vi "FA ForceAndMoments.vi"() -> ()   [LabVIEW 2016, in "M1M3SupportEUI_Views.lvlib"]
uses:
  M1M3SupportEUI_Views.lvlib
  Model/Model.lvclass
  Typedefs/FA Data And Events.ctl
  SALLV_m1m3/DataTypes/ForceActuatorData.ctl
  SALLV_m1m3/DataTypes/logevent_ForceActuatorForceWarning.ctl
  SALLV_m1m3/DataTypes/logevent_ForceActuatorInfo.ctl
  SALLV_m1m3/DataTypes/logevent_ForceActuatorState.ctl
  SALLV_m1m3/DataTypes/logevent_ForceActuatorWarning.ctl
  SALLV_m1m3/DataTypes/logevent_AppliedAberrationForces.ctl
  SALLV_m1m3/DataTypes/logevent_AppliedAccelerationForces.ctl
  SALLV_m1m3/DataTypes/logevent_AppliedActiveOpticForces.ctl
  SALLV_m1m3/DataTypes/logevent_AppliedAzimuthForces.ctl
  SALLV_m1m3/DataTypes/logevent_AppliedBalanceForces.ctl
  SALLV_m1m3/DataTypes/logevent_AppliedCylinderForces.ctl
  SALLV_m1m3/DataTypes/logevent_AppliedElevationForces.ctl
  SALLV_m1m3/DataTypes/logevent_AppliedForces.ctl
  SALLV_m1m3/DataTypes/logevent_AppliedOffsetForces.ctl
  SALLV_m1m3/DataTypes/logevent_AppliedStaticForces.ctl
  SALLV_m1m3/DataTypes/logevent_AppliedThermalForces.ctl
  SALLV_m1m3/DataTypes/logevent_AppliedVelocityForces.ctl
  SALLV_m1m3/DataTypes/logevent_RejectedAberrationForces.ctl
  SALLV_m1m3/DataTypes/logevent_RejectedAccelerationForces.ctl
  SALLV_m1m3/DataTypes/logevent_RejectedActiveOpticForces.ctl
  SALLV_m1m3/DataTypes/logevent_RejectedAzimuthForces.ctl
  SALLV_m1m3/DataTypes/logevent_RejectedBalanceForces.ctl
  SALLV_m1m3/DataTypes/logevent_RejectedCylinderForces.ctl
  SALLV_m1m3/DataTypes/logevent_RejectedElevationForces.ctl
  SALLV_m1m3/DataTypes/logevent_RejectedForces.ctl
  SALLV_m1m3/DataTypes/logevent_RejectedOffsetForces.ctl
  SALLV_m1m3/DataTypes/logevent_RejectedStaticForces.ctl
  SALLV_m1m3/DataTypes/logevent_RejectedThermalForces.ctl
  SALLV_m1m3/DataTypes/logevent_RejectedVelocityForces.ctl
  M1M3 Support Events/M1M3 Support Events.lvclass/M1M3 Support Events.ctl
  M1M3 Support Events/M1M3 Support Events.lvclass
  <vilib>/Utility/Data Type/NI_Data Type.lvlib
  SALLV_m1m3/SALLV_m1m3.lvlib
  Typedefs/M1M3SupportEUI_TypeDefs.lvlib
panel:
  out "Any Secondary Axis Following Error Warning":bool
  out "Any Primary Axis Following Error Warning":bool
  out "Any Secondary Axis Measured Force Warning":bool
  out "Any Primary Axis Measured Force Warning":bool
  out "Any Force Warning":bool
  out "Support %":sgl format="%_4f"
  out "Balance Forces Applied":bool
  out "Acceleration Forces Applied":bool
  out "Offset Forces Applied":bool
  out "Aberration Forces Applied":bool
  out "Active Optic Forces Applied":bool
  out "Velocity Forces Applied":bool
  out "Thermal Forces Applied":bool
  out "Azimuth Forces Applied":bool
  out "Elevation Forces Applied":bool
  out "Static Forces Applied":bool
  out "Slew Flag":bool
  out "Any Broadcast Counter Warning":bool
  out "Any ILC Fault":bool
  out "Any Mezzanine Application CRC Missing":bool
  out "Any Mezzanine Application Missing":bool
  out "Any Mezzanine Backup Calibration Error":bool
  out "Any Mezzanine Event Trap Reset":bool
  out "Any Mezzanine Main Calibration Error":bool
  out "Any Mezzanine Current Amp 2 Fault":bool
  out "Any Mezzanine Unique Id CRC Error":bool
  out "Any Mezzanine Current Amp 1 Fault":bool
  out "Any Mezzanine Power Fault":bool
  out "Any Aux Power Fault":bool
  out "Any SSR Power Fault":bool
  out "Any Event Trap Reset":bool
  out "Any Brown Out":bool
  out "Any Watchdog Reset":bool
  out "Any One Wire 2 Mismatch":bool
  out "Any One Wire 1 Mismatch":bool
  out "Any One Wire Missing":bool
  out "Any Application CRC Missing":bool
  out "Any Application Missing":bool
  out "Any Application Type Mismatch":bool
  out "Any Unique Id CRC Error":bool
  out "Any Mezzanine Bootloader Active":bool
  out "Any Mezzanine Error":bool
  out "Any Backup Calibration Error":bool
  out "Any Main Calibration Error":bool
  out "Any Fault Override":bool
  out "Any Minor Fault":bool
  out "Any Major Fault":bool
  out "Any Warning":bool
  out "Timestamp":timestamp
  out "Force Magnitude":sgl format="%_8f"
  out "Mx":sgl format="%_8f"
  out "My":sgl format="%_8f"
  out "Mz":sgl format="%_8f"
  out "Fz":sgl format="%_8f"
  out "Fy":sgl format="%_8f"
  out "Fx":sgl format="%_8f"
  in  "FA Data And Events":T1 {"ForceActuatorData"."Timestamp" format="%#_14f"}
  in  "Data Type":string(combo)
  in  "Model in":refnum<class "Model.lvclass">
  # "FA Errors (with Forces and Moments)"
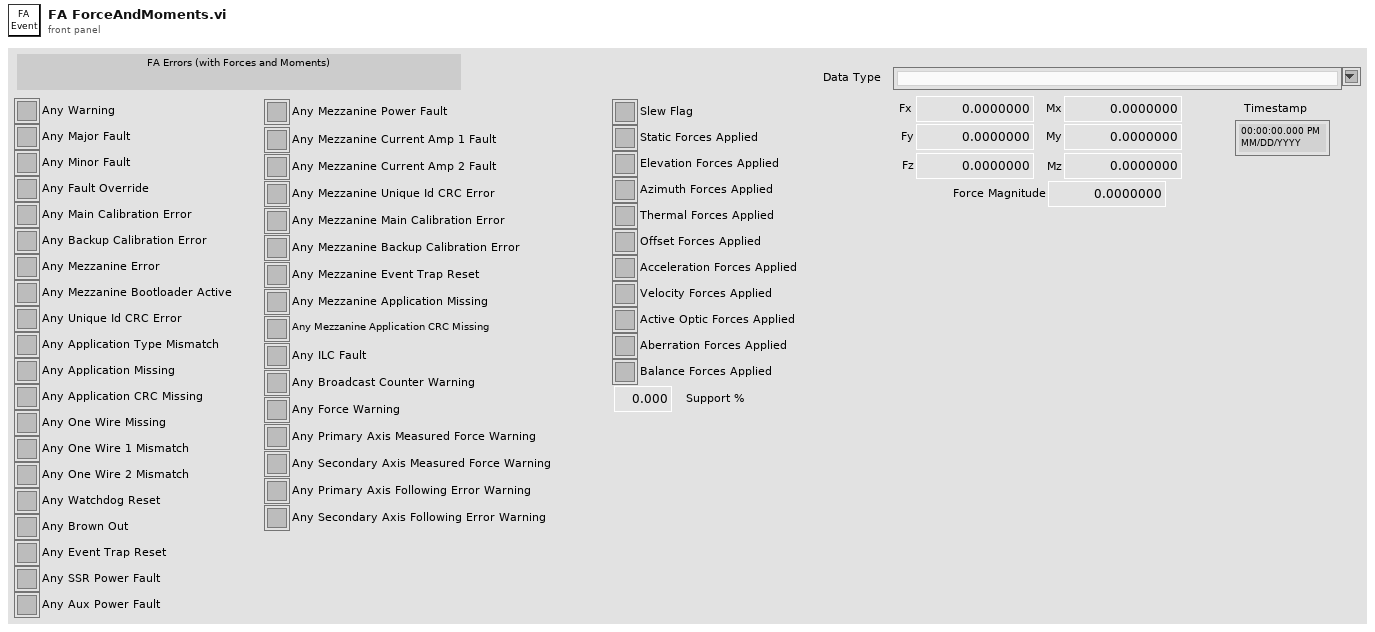
[diagram p1: front panel]
types:
  T1 = typedef "M1M3SupportEUI_TypeDefs.lvlib/FA Data And Events.ctl" = cluster{"ForceActuatorData":T2, "logevent_ForceActuatorForceWarning":T3, "logevent_ForceActuatorInfo":T4, "logevent_ForceActuatorState":T5, "logevent_ForceActuatorWarning":T6, "logevent_AppliedAberrationForces":T7, "logevent_AppliedAccelerationForces":T8, "logevent_AppliedActiveOpticForces":T9, "logevent_AppliedAzimuthForces":T10, "logevent_AppliedBalanceForces":T11, "logevent_AppliedCylinderForces":T12, "logevent_AppliedElevationForces":T13, "logevent_AppliedForces":T14, "logevent_AppliedOffsetForces":T15, "logevent_AppliedStaticForces":T16, "logevent_AppliedThermalForces":T17, "logevent_AppliedVelocityForces":T18, "logevent_RejectedAberrationForces":T19, "logevent_RejectedAccelerationForces":T20, "logevent_RejectedActiveOpticForces":T21, "logevent_RejectedAzimuthForces":T22, "logevent_RejectedBalanceForces":T23, "logevent_RejectedCylinderForces":T24, "logevent_RejectedElevationForces":T25, "logevent_RejectedForces":T26, "logevent_RejectedOffsetForces":T27, "logevent_RejectedStaticForces":T28, "logevent_RejectedThermalForces":T29, "logevent_RejectedVelocityForces":T30}
  T2 = typedef "SALLV_m1m3.lvlib/ForceActuatorData.ctl" = cluster{"Timestamp":dbl, "PrimaryCylinderForce[156]":sgl[], "SecondaryCylinderForce[112]":sgl[], "XForce[12]":sgl[], "YForce[100]":sgl[], "ZForce[156]":sgl[], "Fx":sgl, "Fy":sgl, "Fz":sgl, "Mx":sgl, "My":sgl, "Mz":sgl, "ForceMagnitude":sgl}
  T3 = typedef "SALLV_m1m3.lvlib/logevent_ForceActuatorForceWarning.ctl" = cluster{"Timestamp":dbl, "AnyWarning":bool, "AnyPrimaryAxisMeasuredForceWarning":bool, "PrimaryAxisMeasuredForceWarning[156]":bool[], "AnySecondaryAxisMeasuredForceWarning":bool, "SecondaryAxisMeasuredForceWarning[156]":bool[], "AnyPrimaryAxisFollowingErrorWarning":bool, "PrimaryAxisFollowingErrorWarning[156]":bool[], "AnySecondaryAxisFollowingErrorWarning":bool, "SecondaryAxisFollowingErrorWarning[156]":bool[], "priority":i32}
  T4 = typedef "SALLV_m1m3.lvlib/logevent_ForceActuatorInfo.ctl" = cluster{"Timestamp":dbl, "ReferenceId[156]":i16[], "XDataReferenceId[12]":i16[], "YDataReferenceId[100]":i16[], "ZDataReferenceId[156]":i16[], "ActuatorType[156]":i16[], "ActuatorOrientation[156]":i16[], "ModbusSubnet[156]":i16[], "ModbusAddress[156]":i16[], "XPosition[156]":sgl[], "YPosition[156]":sgl[], "ZPosition[156]":sgl[], "ILCUniqueId[156]":i64[], "ILCApplicationType[156]":i16[], "NetworkNodeType[156]":i16[], "ILCSelectedOptions[156]":i16[], "NetworkNodeOptions[156]":i16[], "MajorRevision[156]":i16[], "MinorRevision[156]":i16[], "ADCScanRate[156]":i16[], "MainPrimaryCylinderCoefficient[156]":sgl[], "MainSecondaryCylinderCoefficient[156]":sgl[], "MainPrimaryCylinderLoadCellOffset[156]":sgl[], "MainSecondaryCylinderLoadCellOffset[156]":sgl[], "MainPrimaryCylinderLoadCellSensitivity[156]":sgl[], "MainSecondaryCylinderLoadCellSensitivity[156]":sgl[], "BackupPrimaryCylinderCoefficient[156]":sgl[], "BackupSecondaryCylinderCoefficient[156]":sgl[], "BackupPrimaryCylinderLoadCellOffset[156]":sgl[], "BackupSecondaryCylinderLoadCellOffset[156]":sgl[], "BackupPrimaryCylinderLoadCellSensitivity[156]":sgl[], "BackupSecondaryCylinderLoadCellSensitivity[156]":sgl[], "MezzaninePrimaryCylinderGain[156]":sgl[], "MezzanineSecondaryCylinderGain[156]":sgl[], "MezzanineUniqueId[156]":i64[], "MezzanineFirmwareType[156]":i16[], "MezzanineMajorRevision[156]":i16[], "MezzanineMinorRevision[156]":i16[], "priority":i32}
  T5 = typedef "SALLV_m1m3.lvlib/logevent_ForceActuatorState.ctl" = cluster{"Timestamp":dbl, "ILCState[156]":i16[], "SlewFlag":bool, "StaticForcesApplied":bool, "ElevationForcesApplied":bool, "AzimuthForcesApplied":bool, "ThermalForcesApplied":bool, "OffsetForcesApplied":bool, "AccelerationForcesApplied":bool, "VelocityForcesApplied":bool, "ActiveOpticForcesApplied":bool, "AberrationForcesApplied":bool, "BalanceForcesApplied":bool, "SupportPercentage":sgl, "priority":i32}
  T6 = typedef "SALLV_m1m3.lvlib/logevent_ForceActuatorWarning.ctl" = cluster{"Timestamp":dbl, "AnyWarning":bool, "AnyMajorFault":bool, "MajorFault[156]":bool[], "AnyMinorFault":bool, "MinorFault[156]":bool[], "AnyFaultOverride":bool, "FaultOverride[156]":bool[], "AnyMainCalibrationError":bool, "MainCalibrationError[156]":bool[], "AnyBackupCalibrationError":bool, "BackupCalibrationError[156]":bool[], "AnyMezzanineError":bool, "MezzanineError[156]":bool[], "AnyMezzanineBootloaderActive":bool, "MezzanineBootloaderActive[156]":bool[], "AnyUniqueIdCRCError":bool, "UniqueIdCRCError[156]":bool[], "AnyApplicationTypeMismatch":bool, "ApplicationTypeMismatch[156]":bool[], "AnyApplicationMissing":bool, "ApplicationMissing[156]":bool[], "AnyApplicationCRCMismatch":bool, "ApplicationCRCMismatch[156]":bool[], "AnyOneWireMissing":bool, "OneWireMissing[156]":bool[], "AnyOneWire1Mismatch":bool, "OneWire1Mismatch[156]":bool[], "AnyOneWire2Mismatch":bool, "OneWire2Mismatch[156]":bool[], "AnyWatchdogReset":bool, "WatchdogReset[156]":bool[], "AnyBrownOut":bool, "BrownOut[156]":bool[], "AnyEventTrapReset":bool, "EventTrapReset[156]":bool[], "AnySSRPowerFault":bool, "SSRPowerFault[156]":bool[], "AnyAuxPowerFault":bool, "AuxPowerFault[156]":bool[], "AnyMezzaninePowerFault":bool, "MezzaninePowerFault[156]":bool[], "AnyMezzanineCurrentAmp1Fault":bool, "MezzanineCurrentAmp1Fault[156]":bool[], "AnyMezzanineCurrentAmp2Fault":bool, "MezzanineCurrentAmp2Fault[156]":bool[], "AnyMezzanineUniqueIdCRCError":bool, "MezzanineUniqueIdCRCError[156]":bool[], "AnyMezzanineMainCalibrationError":bool, "MezzanineMainCalibrationError[156]":bool[], "AnyMezzanineBackupCalibrationError":bool, "MezzanineBackupCalibrationError[156]":bool[], "AnyMezzanineEventTrapReset":bool, "MezzanineEventTrapReset[156]":bool[], "AnyMezzanineApplicationMissing":bool, "MezzanineApplicationMissing[156]":bool[], "AnyMezzanineApplicationCRCMismatch":bool, "MezzanineApplicationCRCMismatch[156]":bool[], "AnyILCFault":bool, "ILCFault[156]":bool[], "AnyBroadcastCounterWarning":bool, "BroadcastCounterWarning[156]":bool[], "priority":i32}
  T7 = typedef "SALLV_m1m3.lvlib/logevent_AppliedAberrationForces.ctl" = cluster{"Timestamp":dbl, "ZForces[156]":sgl[], "Fz":sgl, "Mx":sgl, "My":sgl, "priority":i32}
  T8 = typedef "SALLV_m1m3.lvlib/logevent_AppliedAccelerationForces.ctl" = cluster{"Timestamp":dbl, "XForces[12]":sgl[], "YForces[100]":sgl[], "ZForces[156]":sgl[], "Fx":sgl, "Fy":sgl, "Fz":sgl, "Mx":sgl, "My":sgl, "Mz":sgl, "ForceMagnitude":sgl, "priority":i32}
  T9 = typedef "SALLV_m1m3.lvlib/logevent_AppliedActiveOpticForces.ctl" = cluster{"Timestamp":dbl, "ZForces[156]":sgl[], "Fz":sgl, "Mx":sgl, "My":sgl, "priority":i32}
  T10 = typedef "SALLV_m1m3.lvlib/logevent_AppliedAzimuthForces.ctl" = cluster{"Timestamp":dbl, "XForces[12]":sgl[], "YForces[100]":sgl[], "ZForces[156]":sgl[], "Fx":sgl, "Fy":sgl, "Fz":sgl, "Mx":sgl, "My":sgl, "Mz":sgl, "ForceMagnitude":sgl, "priority":i32}
  T11 = typedef "SALLV_m1m3.lvlib/logevent_AppliedBalanceForces.ctl" = cluster{"Timestamp":dbl, "XForces[12]":sgl[], "YForces[100]":sgl[], "ZForces[156]":sgl[], "Fx":sgl, "Fy":sgl, "Fz":sgl, "Mx":sgl, "My":sgl, "Mz":sgl, "ForceMagnitude":sgl, "priority":i32}
  T12 = typedef "SALLV_m1m3.lvlib/logevent_AppliedCylinderForces.ctl" = cluster{"Timestamp":dbl, "SecondaryCylinderForces[112]":i32[], "PrimaryCylinderForces[156]":i32[], "priority":i32}
  T13 = typedef "SALLV_m1m3.lvlib/logevent_AppliedElevationForces.ctl" = cluster{"Timestamp":dbl, "XForces[12]":sgl[], "YForces[100]":sgl[], "ZForces[156]":sgl[], "Fx":sgl, "Fy":sgl, "Fz":sgl, "Mx":sgl, "My":sgl, "Mz":sgl, "ForceMagnitude":sgl, "priority":i32}
  T14 = typedef "SALLV_m1m3.lvlib/logevent_AppliedForces.ctl" = cluster{"Timestamp":dbl, "XForces[12]":sgl[], "YForces[100]":sgl[], "ZForces[156]":sgl[], "Fx":sgl, "Fy":sgl, "Fz":sgl, "Mx":sgl, "My":sgl, "Mz":sgl, "ForceMagnitude":sgl, "priority":i32}
  T15 = typedef "SALLV_m1m3.lvlib/logevent_AppliedOffsetForces.ctl" = cluster{"Timestamp":dbl, "XForces[12]":sgl[], "YForces[100]":sgl[], "ZForces[156]":sgl[], "Fx":sgl, "Fy":sgl, "Fz":sgl, "Mx":sgl, "My":sgl, "Mz":sgl, "ForceMagnitude":sgl, "priority":i32}
  T16 = typedef "SALLV_m1m3.lvlib/logevent_AppliedStaticForces.ctl" = cluster{"Timestamp":dbl, "XForces[12]":sgl[], "YForces[100]":sgl[], "ZForces[156]":sgl[], "Fx":sgl, "Fy":sgl, "Fz":sgl, "Mx":sgl, "My":sgl, "Mz":sgl, "ForceMagnitude":sgl, "priority":i32}
  T17 = typedef "SALLV_m1m3.lvlib/logevent_AppliedThermalForces.ctl" = cluster{"Timestamp":dbl, "XForces[12]":sgl[], "YForces[100]":sgl[], "ZForces[156]":sgl[], "Fx":sgl, "Fy":sgl, "Fz":sgl, "Mx":sgl, "My":sgl, "Mz":sgl, "ForceMagnitude":sgl, "priority":i32}
  T18 = typedef "SALLV_m1m3.lvlib/logevent_AppliedVelocityForces.ctl" = cluster{"Timestamp":dbl, "XForces[12]":sgl[], "YForces[100]":sgl[], "ZForces[156]":sgl[], "Fx":sgl, "Fy":sgl, "Fz":sgl, "Mx":sgl, "My":sgl, "Mz":sgl, "ForceMagnitude":sgl, "priority":i32}
  T19 = typedef "SALLV_m1m3.lvlib/logevent_RejectedAberrationForces.ctl" = cluster{"Timestamp":dbl, "ZForces[156]":sgl[], "Fz":sgl, "Mx":sgl, "My":sgl, "priority":i32}
  T20 = typedef "SALLV_m1m3.lvlib/logevent_RejectedAccelerationForces.ctl" = cluster{"Timestamp":dbl, "XForces[12]":sgl[], "YForces[100]":sgl[], "ZForces[156]":sgl[], "Fx":sgl, "Fy":sgl, "Fz":sgl, "Mx":sgl, "My":sgl, "Mz":sgl, "ForceMagnitude":sgl, "priority":i32}
  T21 = typedef "SALLV_m1m3.lvlib/logevent_RejectedActiveOpticForces.ctl" = cluster{"Timestamp":dbl, "ZForces[156]":sgl[], "Fz":sgl, "Mx":sgl, "My":sgl, "priority":i32}
  T22 = typedef "SALLV_m1m3.lvlib/logevent_RejectedAzimuthForces.ctl" = cluster{"Timestamp":dbl, "XForces[12]":sgl[], "YForces[100]":sgl[], "ZForces[156]":sgl[], "Fx":sgl, "Fy":sgl, "Fz":sgl, "Mx":sgl, "My":sgl, "Mz":sgl, "ForceMagnitude":sgl, "priority":i32}
  T23 = typedef "SALLV_m1m3.lvlib/logevent_RejectedBalanceForces.ctl" = cluster{"Timestamp":dbl, "XForces[12]":sgl[], "YForces[100]":sgl[], "ZForces[156]":sgl[], "Fx":sgl, "Fy":sgl, "Fz":sgl, "Mx":sgl, "My":sgl, "Mz":sgl, "ForceMagnitude":sgl, "priority":i32}
  T24 = typedef "SALLV_m1m3.lvlib/logevent_RejectedCylinderForces.ctl" = cluster{"Timestamp":dbl, "SecondaryCylinderForces[112]":i32[], "PrimaryCylinderForces[156]":i32[], "priority":i32}
  T25 = typedef "SALLV_m1m3.lvlib/logevent_RejectedElevationForces.ctl" = cluster{"Timestamp":dbl, "XForces[12]":sgl[], "YForces[100]":sgl[], "ZForces[156]":sgl[], "Fx":sgl, "Fy":sgl, "Fz":sgl, "Mx":sgl, "My":sgl, "Mz":sgl, "ForceMagnitude":sgl, "priority":i32}
  T26 = typedef "SALLV_m1m3.lvlib/logevent_RejectedForces.ctl" = cluster{"Timestamp":dbl, "XForces[12]":sgl[], "YForces[100]":sgl[], "ZForces[156]":sgl[], "Fx":sgl, "Fy":sgl, "Fz":sgl, "Mx":sgl, "My":sgl, "Mz":sgl, "ForceMagnitude":sgl, "priority":i32}
  T27 = typedef "SALLV_m1m3.lvlib/logevent_RejectedOffsetForces.ctl" = cluster{"Timestamp":dbl, "XForces[12]":sgl[], "YForces[100]":sgl[], "ZForces[156]":sgl[], "Fx":sgl, "Fy":sgl, "Fz":sgl, "Mx":sgl, "My":sgl, "Mz":sgl, "ForceMagnitude":sgl, "priority":i32}
  T28 = typedef "SALLV_m1m3.lvlib/logevent_RejectedStaticForces.ctl" = cluster{"Timestamp":dbl, "XForces[12]":sgl[], "YForces[100]":sgl[], "ZForces[156]":sgl[], "Fx":sgl, "Fy":sgl, "Fz":sgl, "Mx":sgl, "My":sgl, "Mz":sgl, "ForceMagnitude":sgl, "priority":i32}
  T29 = typedef "SALLV_m1m3.lvlib/logevent_RejectedThermalForces.ctl" = cluster{"Timestamp":dbl, "XForces[12]":sgl[], "YForces[100]":sgl[], "ZForces[156]":sgl[], "Fx":sgl, "Fy":sgl, "Fz":sgl, "Mx":sgl, "My":sgl, "Mz":sgl, "ForceMagnitude":sgl, "priority":i32}
  T30 = typedef "SALLV_m1m3.lvlib/logevent_RejectedVelocityForces.ctl" = cluster{"Timestamp":dbl, "XForces[12]":sgl[], "YForces[100]":sgl[], "ZForces[156]":sgl[], "Fx":sgl, "Fy":sgl, "Fz":sgl, "Mx":sgl, "My":sgl, "Mz":sgl, "ForceMagnitude":sgl, "priority":i32}
  T31 = typedef "M1M3SupportEUI_TypeDefs.lvlib/M1M3 Support Events.ctl" = cluster{"Inclinometer  Data":refnum<user-event>, "IMS Data":refnum<user-event>, "SAL Connected":refnum<user-event>, "Accelerometer Data":refnum<user-event>, "OuterLoop Data":refnum<user-event>, "ErrorCode Event":refnum<user-event>, "InterlockStatus Event":refnum<user-event>, "InterlockWarning Event":refnum<user-event>, "Gyro Data":refnum<user-event>, "HP Actuator Info Event":refnum<user-event>, " FA Info Event":refnum<user-event>, "HP Monitor Info Event":refnum<user-event>, "FA Data":refnum<user-event>, "HP Actuator data":refnum<user-event>, "HP Monitor data":refnum<user-event>, "Air Supply Status Event":refnum<user-event>, "Air Supply Warning Event":refnum<user-event>, "Power Data":refnum<user-event>, "PID Data":refnum<user-event>, "PID Info Event":refnum<user-event>, "Power Status Event":refnum<user-event>, "Power Supply Status Event":refnum<user-event>, "Power Warning Event":refnum<user-event>, "Summary State Event":refnum<user-event>, "Detailed State Event":refnum<user-event>, "FA Force Warning Event":refnum<user-event>, "FA Warning Event":refnum<user-event>, "FA State Event":refnum<user-event>, "Applied AberrationForces Event":refnum<user-event>, "Applied Acceleration Forcces Event":refnum<user-event>, "Applied Azimuth Forces Event":refnum<user-event>, "Applied Active Optic Forces Event":refnum<user-event>, "Applied Balance Forces Event":refnum<user-event>, "Applied Cylinder Forces Event":refnum<user-event>, "Applied Elevation Forces Event":refnum<user-event>, "Applied Forces Event":refnum<user-event>, "Applied Offset Forces Event":refnum<user-event>, "Applied Static Forces Event":refnum<user-event>, "Applied Thermal Forces Event":refnum<user-event>, "Applied Velocity Forces Event":refnum<user-event>, "Rejected Aberration Force Event":refnum<user-event>, "Rejected Acceleration Forces Event":refnum<user-event>, "Rejected Active Optic Forces Event":refnum<user-event>, "Rejected Azimuth Forces Event":refnum<user-event>, "Rejected Balance Forces Event":refnum<user-event>, "Rejected Cylinder Forces Event":refnum<user-event>, "Rejected Elevation Forces Event":refnum<user-event>, "Rejected Forces Event":refnum<user-event>, "Rejected Offset Forces Event":refnum<user-event>, "Rejected Static Forces Event":refnum<user-event>, "Rejected Thermal Forces Event":refnum<user-event>, "Rejected Velocity Forces Event":refnum<user-event>, "Command Rejection Event":refnum<user-event>, "Setting Verions Event":refnum<user-event>, "Settings Applied Event":refnum<user-event>}
  T32 = typedef "NI_Data Type.lvlib/Data Type.ctl" = enum8{"Invalid Type", "Void", "I8", "I16", "I32", "I64", "U8", "U16", "U32", "U64", "Single Float", "Double Float", "Extended Float", "Single Complex", "Double Complex", "Extended Complex", "Enum U8", "Enum U16", "Enum U32", "Enum U64", "Single Float With Unit", "Double Float With Unit", "Extended Float With Unit", "Single Complex with Unit", "Double Complex with Unit", "Extended Complex with Unit", "Boolean", "String", "Path", "Picture", "Tag", "Array", "Cluster", "Variant", "LV Variant", "Waveform", "Timestamp", "Digital Waveform", "Digital Data", "ExpressData", "Refnum", "External Data", "VI", "Poly VI", "LabVIEW Class Instance", "Fixed Point"}
  T33 = enum16{"", "DetailedState_DetailedStates_DisabledState", "DetailedState_DetailedStates_EnabledState", "DetailedState_DetailedStates_FaultState", "DetailedState_DetailedStates_OfflineState", "DetailedState_DetailedStates_StandbyState", "DetailedState_DetailedStates_ParkedState", "DetailedState_DetailedStates_RaisingState", "DetailedState_DetailedStates_ActiveState", "DetailedState_DetailedStates_LoweringState", "DetailedState_DetailedStates_EngineeringState", "DetailedState_DetailedStates_ParkedEngineeringState", "DetailedState_DetailedStates_RaisingEngineeringState", "DetailedState_DetailedStates_ActiveEngineeringState", "DetailedState_DetailedStates_LoweringEngineeringState", "DetailedState_DetailedStates_LoweringFaultState", "DetailedState_DetailedStates_ProfileHardpointCorrectionState"}
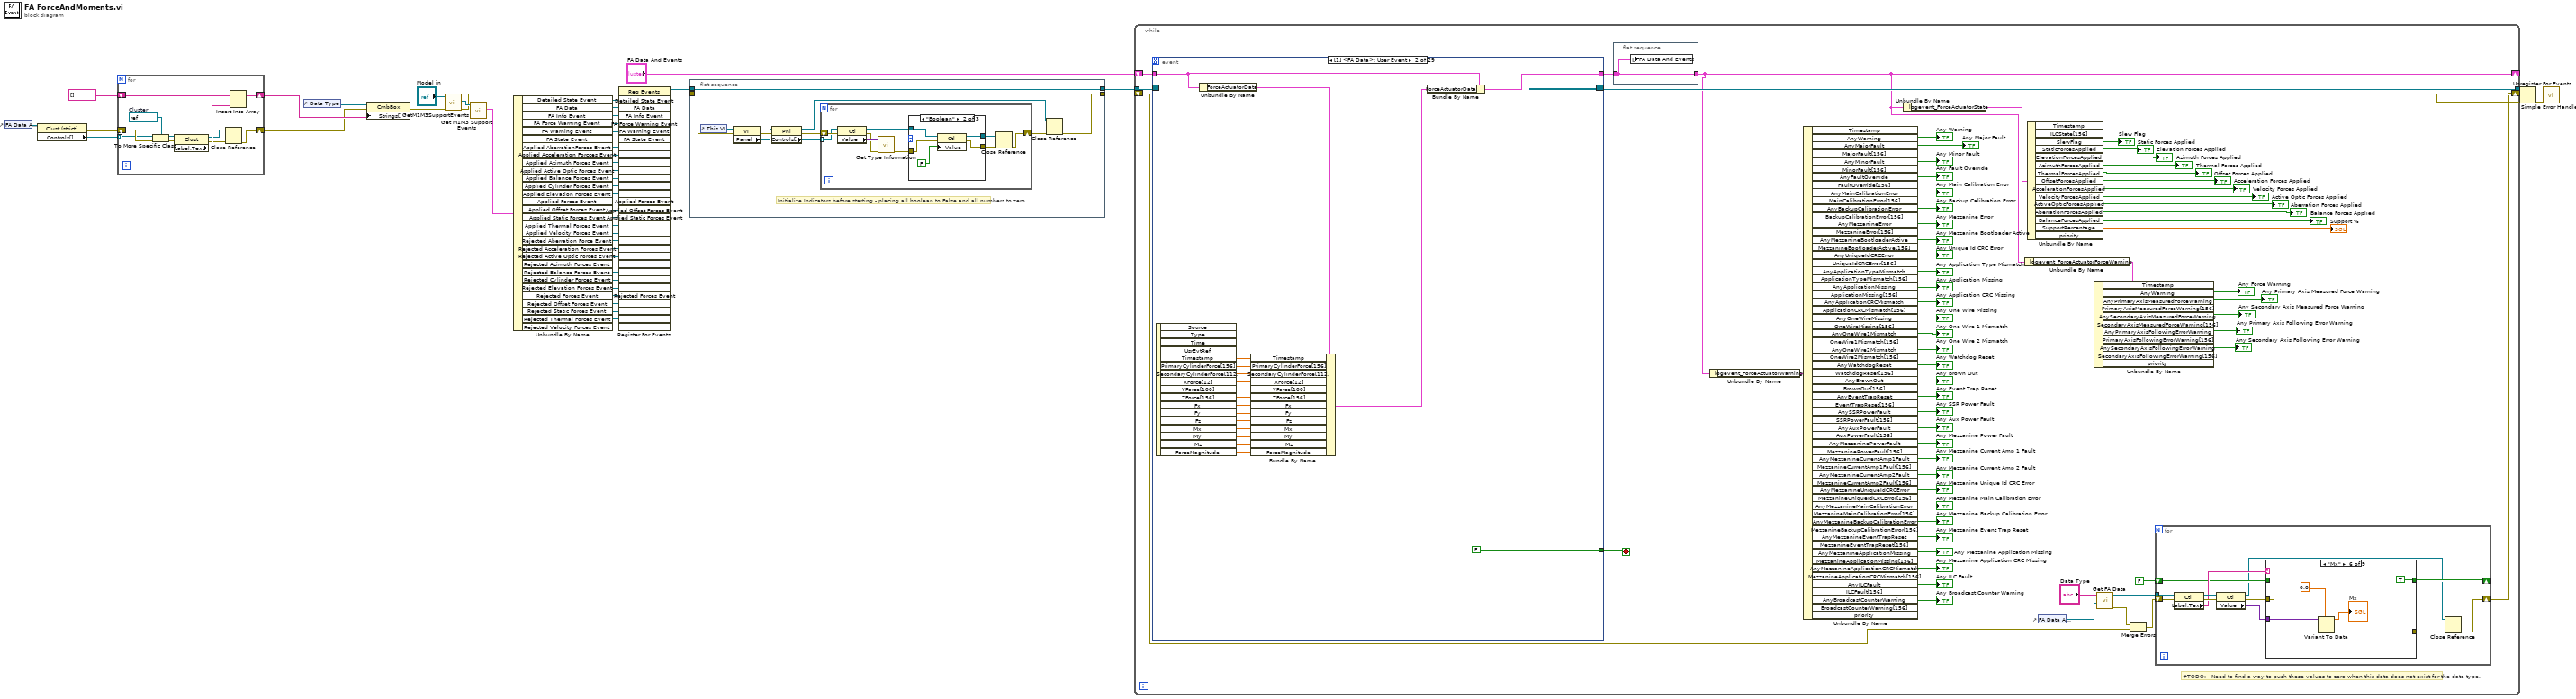
[diagram p0: block diagram]
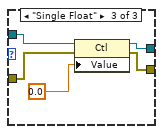
[diagram p3: hidden frame]
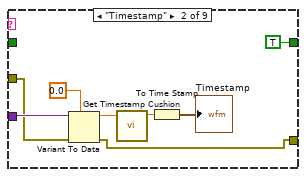
[diagram p5: hidden frame]
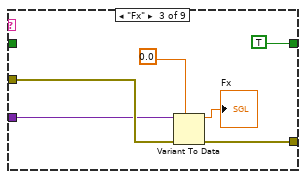
[diagram p6: hidden frame]
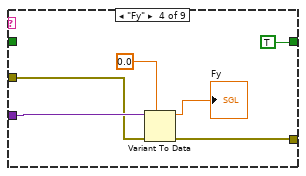
[diagram p7: hidden frame]
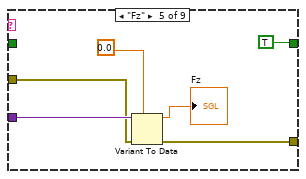
[diagram p8: hidden frame]
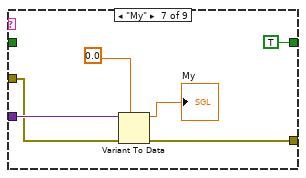
[diagram p9: hidden frame]
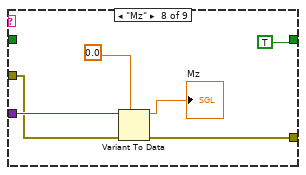
[diagram p10: hidden frame]
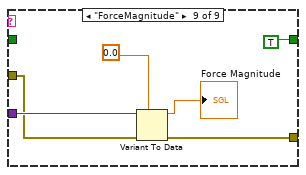
[diagram p11: hidden frame]
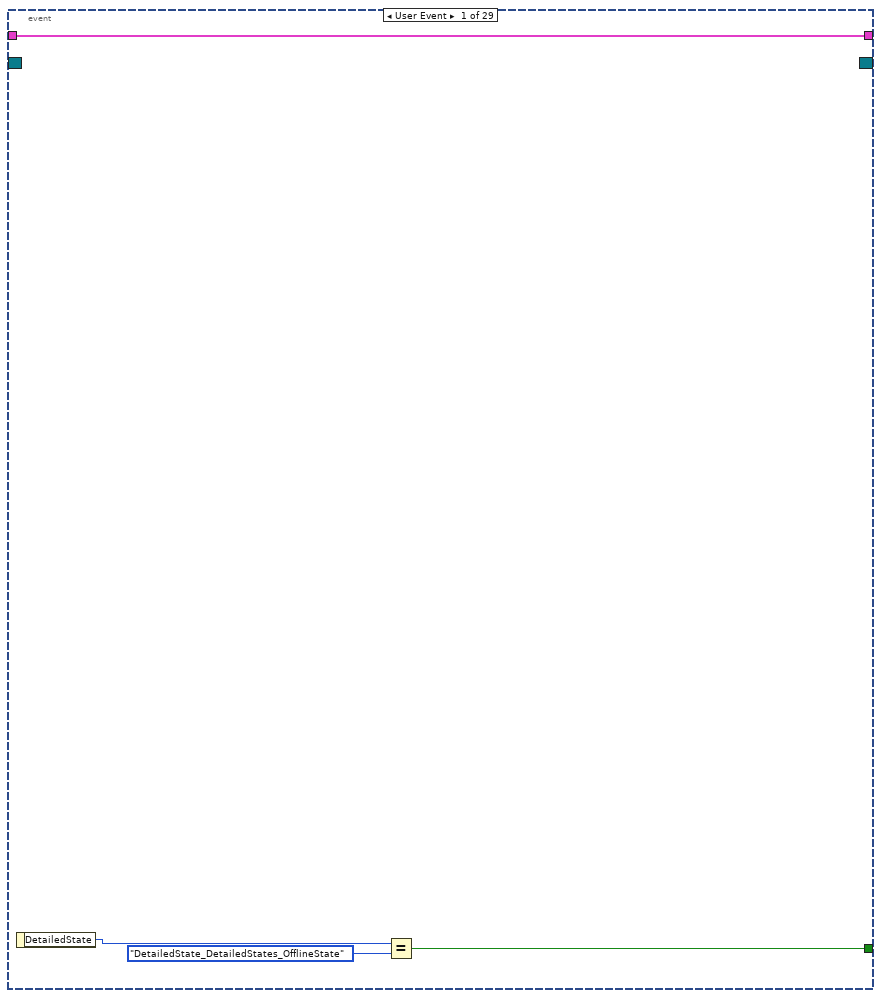
[diagram p12: hidden frame]
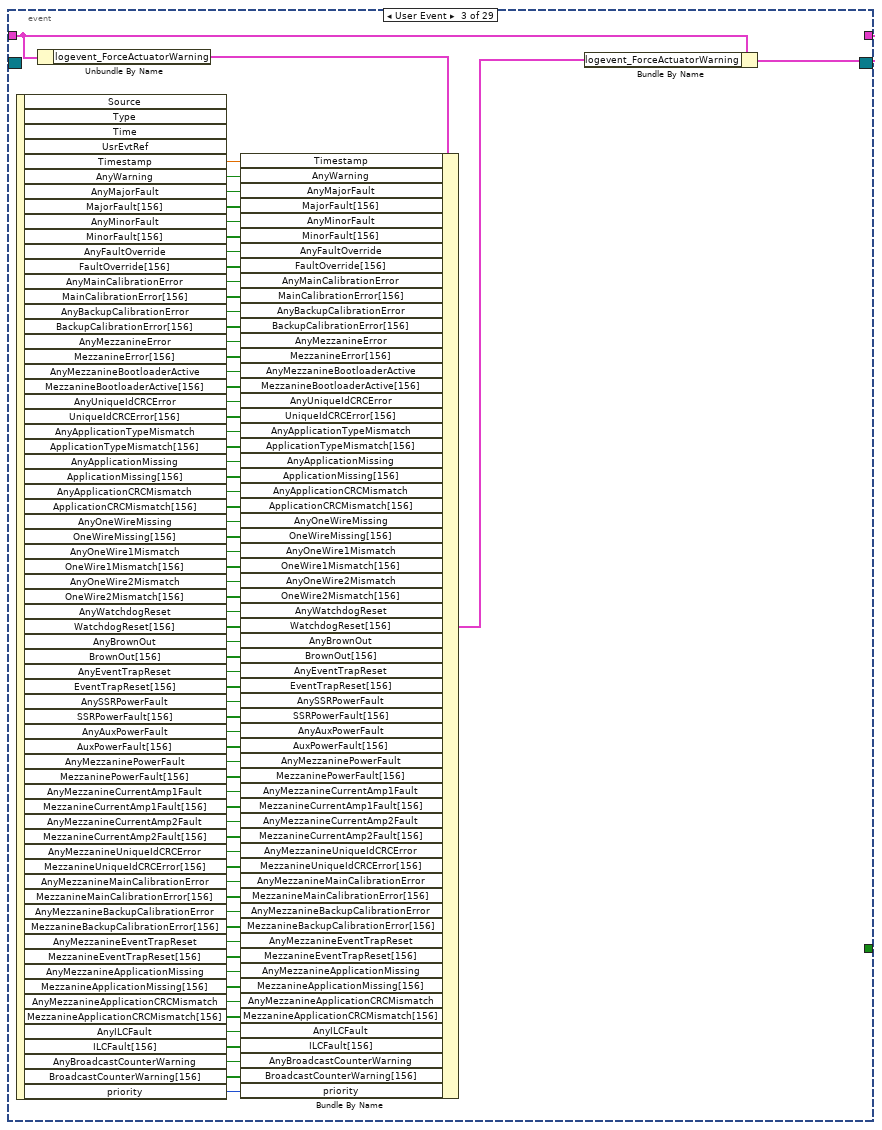
[diagram p13: hidden frame]
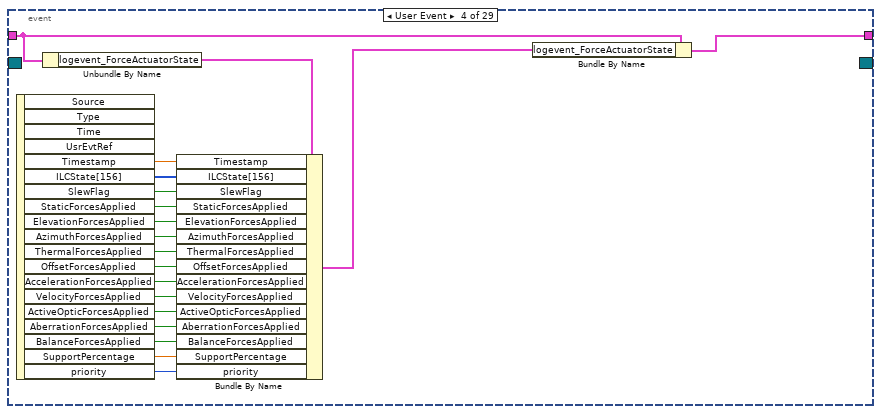
[diagram p14: hidden frame]
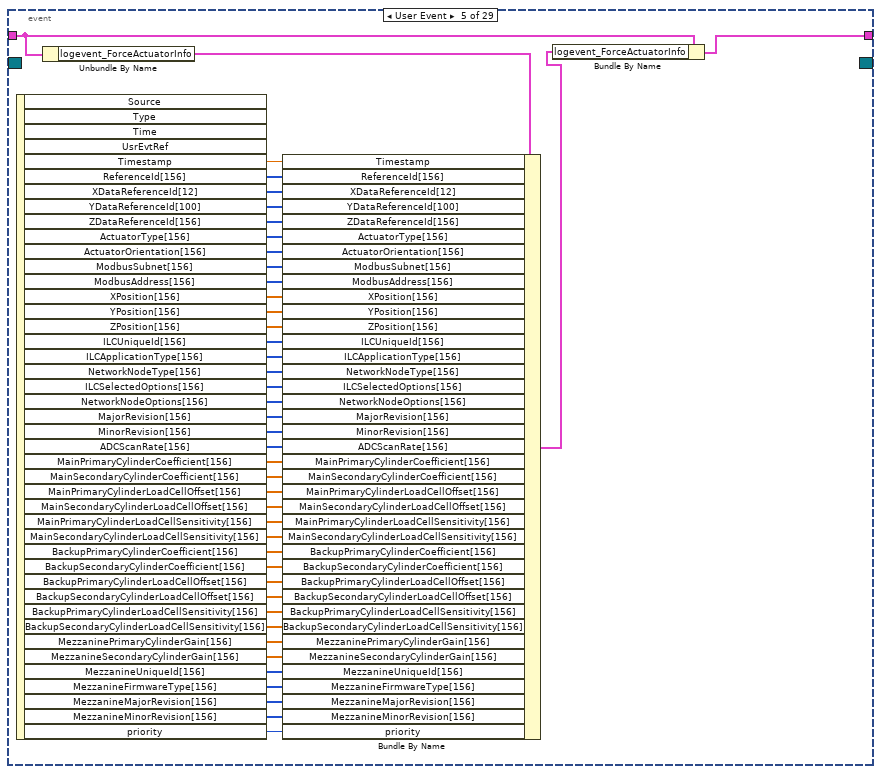
[diagram p15: hidden frame]
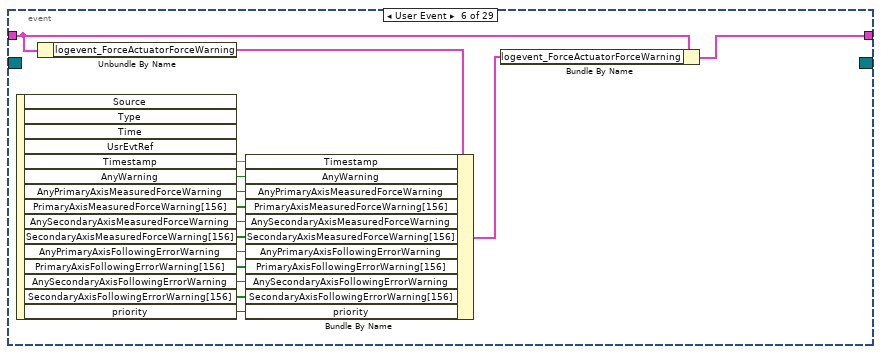
[diagram p16: hidden frame]
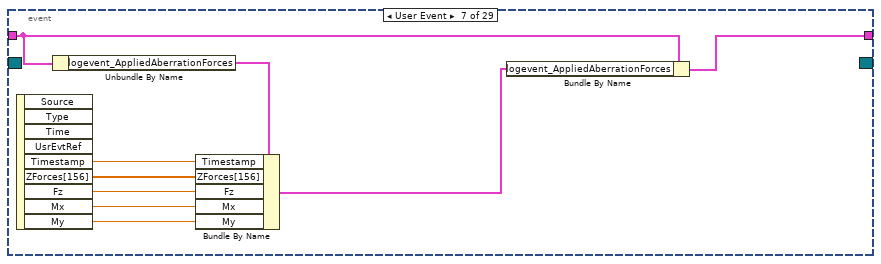
[diagram p17: hidden frame]
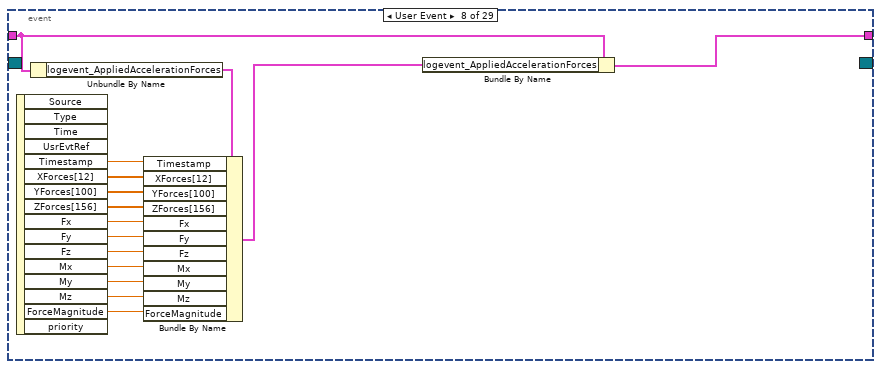
[diagram p18: hidden frame]
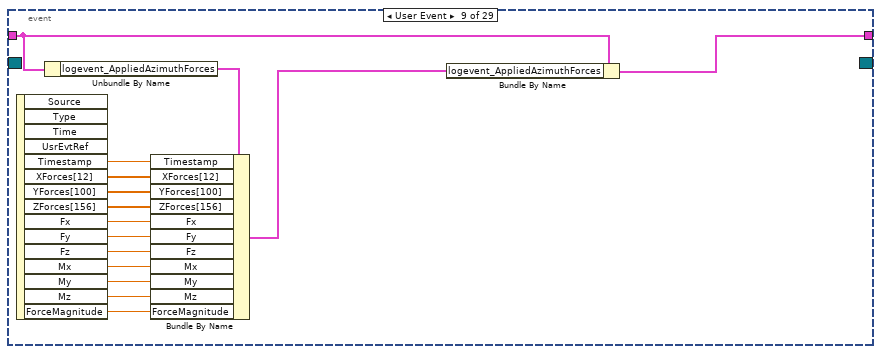
[diagram p19: hidden frame]
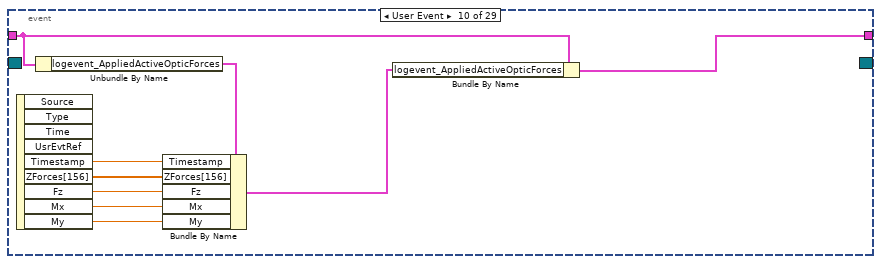
[diagram p20: hidden frame]
diagram:
  n1 = control-ref of="FA Data And Events"() -> (w7:refnum<vi>)
  n2 = property class="Clust (strict)"(reference=w7) -> (error out=w9:errorcluster, "Controls[]"=w10:refnum<vi>[])  [unwired: 1 in, 1 out]
  n3 = for {
    shift-right: [w52] -> w1
    shift-left: w9 -> [w58]
    tunnel: w10 -> [w57] mode=indexing
    shift-right: [w56] -> w8
    shift-left: string[] [] -> [w55]
    w61 = refnum<vi> refnum  # Cluster
    n4 = To More Specific Class(target class=w61, reference=w57, error in=w58) -> (specific class reference=w60:refnum<vi>, error out=w59:errorcluster)
    n5 = property class="Clust"(reference=w60, error in=w59) -> (reference out=w51:refnum<vi>, error out=w53:errorcluster, "Label.Text"=w54:string)
    n6 = Close Reference(reference=w51, error in (no error)=w53) -> (error out=w52:errorcluster)
    n7 = Insert Into Array(array=w55, new element=w54) -> (w56:string[])  [unwired: 1 in]
  }
  n8 = control-ref of="Data Type"() -> (w50:refnum<vi>)
  n9 = property class="CmbBox"(reference=w50, error in=w1, "Strings[]"=w8) -> (error out=w2:errorcluster)  [unwired: 1 out]
  n10 = call "GetM1M3SupportEvents.vi"("error in (no error)"=w2, "Model in"="Model in") -> ("error out"=w17:errorcluster, "M1M3 Support Events out"=w49:refnum<class "M1M3 Support Events.lvclass">)  [unwired: 7 in, 1 out]
  n11 = call "Get M1M3 Support Events.vi"("M1M3 Support Events in"=w49) -> ("M1M3 Support Events"=w16:T31)  [unwired: 9 in, 1 out]
  n12 = Unbundle By Name(w16) -> ("Detailed State Event"=w18:refnum<user-event>, "FA Data"=w19:refnum<user-event>, "FA Info Event"=w20:refnum<user-event>, "FA Force Warning Event"=w21:refnum<user-event>, "FA Warning Event"=w23:refnum<user-event>, "FA State Event"=w22:refnum<user-event>, "Applied AberrationForces Event"=w24:refnum<user-event>, "Applied Acceleration Forcces Event"=w25:refnum<user-event>, "Applied Azimuth Forces Event"=w26:refnum<user-event>, "Applied Active Optic Forces Event"=w27:refnum<user-event>, "Applied Balance Forces Event"=w28:refnum<user-event>, "Applied Cylinder Forces Event"=w29:refnum<user-event>, "Applied Elevation Forces Event"=w30:refnum<user-event>, "Applied Forces Event"=w31:refnum<user-event>, "Applied Offset Forces Event"=w32:refnum<user-event>, "Applied Static Forces Event"=w33:refnum<user-event>, "Applied Thermal Forces Event"=w34:refnum<user-event>, "Applied Velocity Forces Event"=w35:refnum<user-event>, "Rejected Aberration Force Event"=w36:refnum<user-event>, "Rejected Acceleration Forces Event"=w37:refnum<user-event>, "Rejected Active Optic Forces Event"=w38:refnum<user-event>, "Rejected Azimuth Forces Event"=w39:refnum<user-event>, "Rejected Balance Forces Event"=w40:refnum<user-event>, "Rejected Cylinder Forces Event"=w41:refnum<user-event>, "Rejected Elevation Forces Event"=w42:refnum<user-event>, "Rejected Forces Event"=w43:refnum<user-event>, "Rejected Offset Forces Event"=w44:refnum<user-event>, "Rejected Static Forces Event"=w45:refnum<user-event>, "Rejected Thermal Forces Event"=w46:refnum<user-event>, "Rejected Velocity Forces Event"=w47:refnum<user-event>)
  n13 = register-events(error in=w17, w18, w19, w20, w21, w23, w22, w24, w25, w26, w27, w28, w29, w30, w31, w32, w33, w34, w35, w36, w37, w38, w39, w40, w41, w42, w43, w44, w45, w46, w47) -> (reference out=w5:refnum<event-registration>, error out=w4:errorcluster)  [unwired: 1 in]
  n14 = flat-sequence {
    tunnel: [w71] -> w6
    tunnel: w5 -> [w71]
    tunnel: w4 -> [w67]
    tunnel: [w62] -> w3
    frame #0 {
      # "Initialize Indicators before starting - placing all boolean to False and all numbers to zero."
      n15 = control-ref of="This VI"() -> (w70:refnum<vi>)
      n16 = property class="VI"(reference=w70, error in=w67) -> (error out=w69:errorcluster, "Panel"=w68:refnum<vi>)  [unwired: 1 out]
      n17 = property class="Pnl"(reference=w68, error in=w69) -> (reference out=w64:refnum<vi>, error out=w65:errorcluster, "Controls[]"=w66:refnum<vi>[])
      n18 = for {
        tunnel: w66 -> [w80] mode=indexing
        shift-right: [w73] -> w63
        shift-left: w65 -> [w81]
        n19 = property class="Ctl"(reference=w80, error in=w81) -> (reference out=w76:refnum<vi>, error out=w78:errorcluster, "Value"=w79:variant)
        n20 = call <vilib>:"Get Type Information.vi"("error in (no error)"=w78, "Variant"=w79) -> ("error out"=w77:errorcluster, "Type"=w72:T32)  [unwired: 5 in, 3 out]
        n21 = case shown="\"Boolean\"" w72 {
          tunnel: w77 -> [w82 w86 w92]
          tunnel: w76 -> [w83 w88 w93]
          tunnel: [w83 w85 w91] -> w75
          tunnel: [w82 w84 w90] -> w74
          frame "Invalid Type", Default {
          }
          frame "Boolean" {
            n22 = property class="Ctl"(reference=w88, error in=w86, "Value"=FALSE) -> (reference out=w85:refnum<vi>, error out=w84:errorcluster)
          }
          frame "Single Float" {
            n23 = property class="Ctl"(reference=w93, error in=w92, "Value"=sgl 0.0) -> (reference out=w91:refnum<vi>, error out=w90:errorcluster)
          }
        }
        n24 = Close Reference(reference=w75, error in (no error)=w74) -> (error out=w73:errorcluster)
      }
      n25 = Close Reference(reference=w64, error in (no error)=w63) -> (error out=w62:errorcluster)
    }
  }
  n26 = while {
    tunnel: w6 -> [w157]
    tunnel: [w156] -> w15
    shift-right: [w95] -> w14
    shift-left: w3 -> [w96]
    shift-right: [w97] -> _
    shift-left: "FA Data And Events" -> [w158]
    stop <- w155 stop-if-true
    # "#TODO:   Need to find a way to push these values to zero when this data does not exist for the data type."
    n27 = event shown="[1] <FA Data>: User Event" {
      selector: w157 -> [_ _ _ _ _ _ _ _ _ _ _ _ _ _ _ _ _ _ _ _ _ _ _ _ _ _ _ _ _]
      dyn-events: [_ _ _ _ _ _ _ _ _ _ _ _ _ _ _ _ _ _ _ _ _ _ _ _ _ _ _ _ _] -> w156
      timeout: _ -> [_ _ _ _ _ _ _ _ _ _ _ _ _ _ _ _ _ _ _ _ _ _ _ _ _ _ _ _ _]
      tunnel: [w227 FALSE _ _ _ _ _ _ _ _ _ _ _ _ _ _ _ _ _ _ _ _ _ _ _ _ _ _ _] -> w155
      tunnel: w158 -> [w226 w237 w279 w327 w334 w382 w392 w401 w416 w431 w440 w455 w462 w477 w492 w507 w521 w537 w552 w561 w576 w585 w600 w615 w622 w637 w652 w667 w682]
      tunnel: [w226 w235 w278 w325 w333 w381 w390 w399 w414 w429 w438 w453 w460 w475 w490 w505 w520 w535 w550 w559 w574 w583 w598 w613 w620 w635 w650 w665 w680] -> w154
      event User Event {
        n28 = event-data() -> ("DetailedState"=w225:T33)  [unwired: 1 in]
        n29 = Equal?(x=w225, y=T33."DetailedState_DetailedStates_OfflineState") -> (x = y?=w227:bool)
      }
      event User Event {
        n30 = event-data() -> ("Timestamp"=w239:dbl, "PrimaryCylinderForce[156]"=w244:sgl[], "SecondaryCylinderForce[112]"=w243:sgl[], "XForce[12]"=w242:sgl[], "YForce[100]"=w241:sgl[], "ZForce[156]"=w240:sgl[], "Fx"=w234:sgl, "Fy"=w233:sgl, "Fz"=w232:sgl, "Mx"=w231:sgl, "My"=w230:sgl, "Mz"=w229:sgl, "ForceMagnitude"=w228:sgl)  [unwired: 1 in, 4 out]
        n31 = Unbundle By Name(w237) -> ("ForceActuatorData"=w238:T2)
        n32 = Bundle By Name(cluster=w238, "Timestamp"=w239, "PrimaryCylinderForce[156]"=w244, "SecondaryCylinderForce[112]"=w243, "XForce[12]"=w242, "YForce[100]"=w241, "ZForce[156]"=w240, "Fx"=w234, "Fy"=w233, "Fz"=w232, "Mx"=w231, "My"=w230, "Mz"=w229, "ForceMagnitude"=w228) -> (w236:T2)
        n33 = Bundle By Name(cluster=w237, "ForceActuatorData"=w236) -> (w235:T1)
      }
      event User Event {
        n34 = event-data() -> ("Timestamp"=w281:dbl, "AnyWarning"=w276:bool, "AnyMajorFault"=w275:bool, "MajorFault[156]"=w312:bool[], "AnyMinorFault"=w274:bool, "MinorFault[156]"=w311:bool[], "AnyFaultOverride"=w273:bool, "FaultOverride[156]"=w310:bool[], "AnyMainCalibrationError"=w272:bool, "MainCalibrationError[156]"=w309:bool[], "AnyBackupCalibrationError"=w271:bool, "BackupCalibrationError[156]"=w308:bool[], "AnyMezzanineError"=w270:bool, "MezzanineError[156]"=w307:bool[], "AnyMezzanineBootloaderActive"=w269:bool, "MezzanineBootloaderActive[156]"=w306:bool[], "AnyUniqueIdCRCError"=w268:bool, "UniqueIdCRCError[156]"=w305:bool[], "AnyApplicationTypeMismatch"=w267:bool, "ApplicationTypeMismatch[156]"=w304:bool[], "AnyApplicationMissing"=w266:bool, "ApplicationMissing[156]"=w303:bool[], "AnyApplicationCRCMismatch"=w265:bool, "ApplicationCRCMismatch[156]"=w302:bool[], "AnyOneWireMissing"=w264:bool, "OneWireMissing[156]"=w301:bool[], "AnyOneWire1Mismatch"=w263:bool, "OneWire1Mismatch[156]"=w300:bool[], "AnyOneWire2Mismatch"=w262:bool, "OneWire2Mismatch[156]"=w299:bool[], "AnyWatchdogReset"=w261:bool, "WatchdogReset[156]"=w298:bool[], "AnyBrownOut"=w260:bool, "BrownOut[156]"=w297:bool[], "AnyEventTrapReset"=w259:bool, "EventTrapReset[156]"=w296:bool[], "AnySSRPowerFault"=w258:bool, "SSRPowerFault[156]"=w295:bool[], "AnyAuxPowerFault"=w257:bool, "AuxPowerFault[156]"=w294:bool[], "AnyMezzaninePowerFault"=w256:bool, "MezzaninePowerFault[156]"=w293:bool[], "AnyMezzanineCurrentAmp1Fault"=w255:bool, "MezzanineCurrentAmp1Fault[156]"=w292:bool[], "AnyMezzanineCurrentAmp2Fault"=w254:bool, "MezzanineCurrentAmp2Fault[156]"=w291:bool[], "AnyMezzanineUniqueIdCRCError"=w253:bool, "MezzanineUniqueIdCRCError[156]"=w290:bool[], "AnyMezzanineMainCalibrationError"=w252:bool, "MezzanineMainCalibrationError[156]"=w289:bool[], "AnyMezzanineBackupCalibrationError"=w251:bool, "MezzanineBackupCalibrationError[156]"=w288:bool[], "AnyMezzanineEventTrapReset"=w250:bool, "MezzanineEventTrapReset[156]"=w287:bool[], "AnyMezzanineApplicationMissing"=w249:bool, "MezzanineApplicationMissing[156]"=w286:bool[], "AnyMezzanineApplicationCRCMismatch"=w248:bool, "MezzanineApplicationCRCMismatch[156]"=w285:bool[], "AnyILCFault"=w247:bool, "ILCFault[156]"=w284:bool[], "AnyBroadcastCounterWarning"=w246:bool, "BroadcastCounterWarning[156]"=w283:bool[], "priority"=w282:i32)  [unwired: 1 in, 4 out]
        n35 = Unbundle By Name(w279) -> ("logevent_ForceActuatorWarning"=w280:T6)
        n36 = Bundle By Name(cluster=w280, "Timestamp"=w281, "AnyWarning"=w276, "AnyMajorFault"=w275, "MajorFault[156]"=w312, "AnyMinorFault"=w274, "MinorFault[156]"=w311, "AnyFaultOverride"=w273, "FaultOverride[156]"=w310, "AnyMainCalibrationError"=w272, "MainCalibrationError[156]"=w309, "AnyBackupCalibrationError"=w271, "BackupCalibrationError[156]"=w308, "AnyMezzanineError"=w270, "MezzanineError[156]"=w307, "AnyMezzanineBootloaderActive"=w269, "MezzanineBootloaderActive[156]"=w306, "AnyUniqueIdCRCError"=w268, "UniqueIdCRCError[156]"=w305, "AnyApplicationTypeMismatch"=w267, "ApplicationTypeMismatch[156]"=w304, "AnyApplicationMissing"=w266, "ApplicationMissing[156]"=w303, "AnyApplicationCRCMismatch"=w265, "ApplicationCRCMismatch[156]"=w302, "AnyOneWireMissing"=w264, "OneWireMissing[156]"=w301, "AnyOneWire1Mismatch"=w263, "OneWire1Mismatch[156]"=w300, "AnyOneWire2Mismatch"=w262, "OneWire2Mismatch[156]"=w299, "AnyWatchdogReset"=w261, "WatchdogReset[156]"=w298, "AnyBrownOut"=w260, "BrownOut[156]"=w297, "AnyEventTrapReset"=w259, "EventTrapReset[156]"=w296, "AnySSRPowerFault"=w258, "SSRPowerFault[156]"=w295, "AnyAuxPowerFault"=w257, "AuxPowerFault[156]"=w294, "AnyMezzaninePowerFault"=w256, "MezzaninePowerFault[156]"=w293, "AnyMezzanineCurrentAmp1Fault"=w255, "MezzanineCurrentAmp1Fault[156]"=w292, "AnyMezzanineCurrentAmp2Fault"=w254, "MezzanineCurrentAmp2Fault[156]"=w291, "AnyMezzanineUniqueIdCRCError"=w253, "MezzanineUniqueIdCRCError[156]"=w290, "AnyMezzanineMainCalibrationError"=w252, "MezzanineMainCalibrationError[156]"=w289, "AnyMezzanineBackupCalibrationError"=w251, "MezzanineBackupCalibrationError[156]"=w288, "AnyMezzanineEventTrapReset"=w250, "MezzanineEventTrapReset[156]"=w287, "AnyMezzanineApplicationMissing"=w249, "MezzanineApplicationMissing[156]"=w286, "AnyMezzanineApplicationCRCMismatch"=w248, "MezzanineApplicationCRCMismatch[156]"=w285, "AnyILCFault"=w247, "ILCFault[156]"=w284, "AnyBroadcastCounterWarning"=w246, "BroadcastCounterWarning[156]"=w283, "priority"=w282) -> (w277:T6)
        n37 = Bundle By Name(cluster=w279, "logevent_ForceActuatorWarning"=w277) -> (w278:T1)
      }
      event User Event {
        n38 = event-data() -> ("Timestamp"=w329:dbl, "ILCState[156]"=w331:i16[], "SlewFlag"=w324:bool, "StaticForcesApplied"=w323:bool, "ElevationForcesApplied"=w322:bool, "AzimuthForcesApplied"=w321:bool, "ThermalForcesApplied"=w320:bool, "OffsetForcesApplied"=w319:bool, "AccelerationForcesApplied"=w318:bool, "VelocityForcesApplied"=w317:bool, "ActiveOpticForcesApplied"=w316:bool, "AberrationForcesApplied"=w314:bool, "BalanceForcesApplied"=w315:bool, "SupportPercentage"=w313:sgl, "priority"=w330:i32)  [unwired: 1 in, 4 out]
        n39 = Unbundle By Name(w327) -> ("logevent_ForceActuatorState"=w328:T5)
        n40 = Bundle By Name(cluster=w328, "Timestamp"=w329, "ILCState[156]"=w331, "SlewFlag"=w324, "StaticForcesApplied"=w323, "ElevationForcesApplied"=w322, "AzimuthForcesApplied"=w321, "ThermalForcesApplied"=w320, "OffsetForcesApplied"=w319, "AccelerationForcesApplied"=w318, "VelocityForcesApplied"=w317, "ActiveOpticForcesApplied"=w316, "AberrationForcesApplied"=w314, "BalanceForcesApplied"=w315, "SupportPercentage"=w313, "priority"=w330) -> (w326:T5)
        n41 = Bundle By Name(cluster=w327, "logevent_ForceActuatorState"=w326) -> (w325:T1)
      }
      event User Event {
        n42 = event-data() -> ("Timestamp"=w336:dbl, "ReferenceId[156]"=w374:i16[], "XDataReferenceId[12]"=w373:i16[], "YDataReferenceId[100]"=w372:i16[], "ZDataReferenceId[156]"=w371:i16[], "ActuatorType[156]"=w370:i16[], "ActuatorOrientation[156]"=w369:i16[], "ModbusSubnet[156]"=w368:i16[], "ModbusAddress[156]"=w367:i16[], "XPosition[156]"=w366:sgl[], "YPosition[156]"=w365:sgl[], "ZPosition[156]"=w364:sgl[], "ILCUniqueId[156]"=w363:i64[], "ILCApplicationType[156]"=w362:i16[], "NetworkNodeType[156]"=w361:i16[], "ILCSelectedOptions[156]"=w360:i16[], "NetworkNodeOptions[156]"=w359:i16[], "MajorRevision[156]"=w358:i16[], "MinorRevision[156]"=w357:i16[], "ADCScanRate[156]"=w356:i16[], "MainPrimaryCylinderCoefficient[156]"=w355:sgl[], "MainSecondaryCylinderCoefficient[156]"=w354:sgl[], "MainPrimaryCylinderLoadCellOffset[156]"=w353:sgl[], "MainSecondaryCylinderLoadCellOffset[156]"=w352:sgl[], "MainPrimaryCylinderLoadCellSensitivity[156]"=w351:sgl[], "MainSecondaryCylinderLoadCellSensitivity[156]"=w350:sgl[], "BackupPrimaryCylinderCoefficient[156]"=w349:sgl[], "BackupSecondaryCylinderCoefficient[156]"=w348:sgl[], "BackupPrimaryCylinderLoadCellOffset[156]"=w347:sgl[], "BackupSecondaryCylinderLoadCellOffset[156]"=w346:sgl[], "BackupPrimaryCylinderLoadCellSensitivity[156]"=w345:sgl[], "BackupSecondaryCylinderLoadCellSensitivity[156]"=w344:sgl[], "MezzaninePrimaryCylinderGain[156]"=w343:sgl[], "MezzanineSecondaryCylinderGain[156]"=w342:sgl[], "MezzanineUniqueId[156]"=w341:i64[], "MezzanineFirmwareType[156]"=w340:i16[], "MezzanineMajorRevision[156]"=w339:i16[], "MezzanineMinorRevision[156]"=w338:i16[], "priority"=w337:i32)  [unwired: 1 in, 4 out]
        n43 = Unbundle By Name(w334) -> ("logevent_ForceActuatorInfo"=w335:T4)
        n44 = Bundle By Name(cluster=w335, "Timestamp"=w336, "ReferenceId[156]"=w374, "XDataReferenceId[12]"=w373, "YDataReferenceId[100]"=w372, "ZDataReferenceId[156]"=w371, "ActuatorType[156]"=w370, "ActuatorOrientation[156]"=w369, "ModbusSubnet[156]"=w368, "ModbusAddress[156]"=w367, "XPosition[156]"=w366, "YPosition[156]"=w365, "ZPosition[156]"=w364, "ILCUniqueId[156]"=w363, "ILCApplicationType[156]"=w362, "NetworkNodeType[156]"=w361, "ILCSelectedOptions[156]"=w360, "NetworkNodeOptions[156]"=w359, "MajorRevision[156]"=w358, "MinorRevision[156]"=w357, "ADCScanRate[156]"=w356, "MainPrimaryCylinderCoefficient[156]"=w355, "MainSecondaryCylinderCoefficient[156]"=w354, "MainPrimaryCylinderLoadCellOffset[156]"=w353, "MainSecondaryCylinderLoadCellOffset[156]"=w352, "MainPrimaryCylinderLoadCellSensitivity[156]"=w351, "MainSecondaryCylinderLoadCellSensitivity[156]"=w350, "BackupPrimaryCylinderCoefficient[156]"=w349, "BackupSecondaryCylinderCoefficient[156]"=w348, "BackupPrimaryCylinderLoadCellOffset[156]"=w347, "BackupSecondaryCylinderLoadCellOffset[156]"=w346, "BackupPrimaryCylinderLoadCellSensitivity[156]"=w345, "BackupSecondaryCylinderLoadCellSensitivity[156]"=w344, "MezzaninePrimaryCylinderGain[156]"=w343, "MezzanineSecondaryCylinderGain[156]"=w342, "MezzanineUniqueId[156]"=w341, "MezzanineFirmwareType[156]"=w340, "MezzanineMajorRevision[156]"=w339, "MezzanineMinorRevision[156]"=w338, "priority"=w337) -> (w332:T4)
        n45 = Bundle By Name(cluster=w334, "logevent_ForceActuatorInfo"=w332) -> (w333:T1)
      }
      event User Event {
        n46 = event-data() -> ("Timestamp"=w384:dbl, "AnyWarning"=w379:bool, "AnyPrimaryAxisMeasuredForceWarning"=w378:bool, "PrimaryAxisMeasuredForceWarning[156]"=w389:bool[], "AnySecondaryAxisMeasuredForceWarning"=w377:bool, "SecondaryAxisMeasuredForceWarning[156]"=w388:bool[], "AnyPrimaryAxisFollowingErrorWarning"=w376:bool, "PrimaryAxisFollowingErrorWarning[156]"=w387:bool[], "AnySecondaryAxisFollowingErrorWarning"=w375:bool, "SecondaryAxisFollowingErrorWarning[156]"=w386:bool[], "priority"=w385:i32)  [unwired: 1 in, 4 out]
        n47 = Unbundle By Name(w382) -> ("logevent_ForceActuatorForceWarning"=w383:T3)
        n48 = Bundle By Name(cluster=w383, "Timestamp"=w384, "AnyWarning"=w379, "AnyPrimaryAxisMeasuredForceWarning"=w378, "PrimaryAxisMeasuredForceWarning[156]"=w389, "AnySecondaryAxisMeasuredForceWarning"=w377, "SecondaryAxisMeasuredForceWarning[156]"=w388, "AnyPrimaryAxisFollowingErrorWarning"=w376, "PrimaryAxisFollowingErrorWarning[156]"=w387, "AnySecondaryAxisFollowingErrorWarning"=w375, "SecondaryAxisFollowingErrorWarning[156]"=w386, "priority"=w385) -> (w380:T3)
        n49 = Bundle By Name(cluster=w382, "logevent_ForceActuatorForceWarning"=w380) -> (w381:T1)
      }
      event User Event {
        n50 = event-data() -> ("Timestamp"=w397:dbl, "ZForces[156]"=w396:sgl[], "Fz"=w395:sgl, "Mx"=w394:sgl, "My"=w393:sgl)  [unwired: 1 in, 4 out]
        n51 = Unbundle By Name(w392) -> ("logevent_AppliedAberrationForces"=w398:T7)
        n52 = Bundle By Name(cluster=w398, "Timestamp"=w397, "ZForces[156]"=w396, "Fz"=w395, "Mx"=w394, "My"=w393) -> (w391:T7)
        n53 = Bundle By Name(cluster=w392, "logevent_AppliedAberrationForces"=w391) -> (w390:T1)
      }
      event User Event {
        n54 = event-data() -> ("Timestamp"=w412:dbl, "XForces[12]"=w411:sgl[], "YForces[100]"=w410:sgl[], "ZForces[156]"=w409:sgl[], "Fx"=w408:sgl, "Fy"=w407:sgl, "Fz"=w406:sgl, "Mx"=w405:sgl, "My"=w404:sgl, "Mz"=w403:sgl, "ForceMagnitude"=w402:sgl)  [unwired: 1 in, 5 out]
        n55 = Unbundle By Name(w401) -> ("logevent_AppliedAccelerationForces"=w413:T8)
        n56 = Bundle By Name(cluster=w413, "Timestamp"=w412, "XForces[12]"=w411, "YForces[100]"=w410, "ZForces[156]"=w409, "Fx"=w408, "Fy"=w407, "Fz"=w406, "Mx"=w405, "My"=w404, "Mz"=w403, "ForceMagnitude"=w402) -> (w400:T8)
        n57 = Bundle By Name(cluster=w401, "logevent_AppliedAccelerationForces"=w400) -> (w399:T1)
      }
      event User Event {
        n58 = event-data() -> ("Timestamp"=w427:dbl, "XForces[12]"=w426:sgl[], "YForces[100]"=w425:sgl[], "ZForces[156]"=w424:sgl[], "Fx"=w423:sgl, "Fy"=w422:sgl, "Fz"=w421:sgl, "Mx"=w420:sgl, "My"=w419:sgl, "Mz"=w418:sgl, "ForceMagnitude"=w417:sgl)  [unwired: 1 in, 4 out]
        n59 = Unbundle By Name(w416) -> ("logevent_AppliedAzimuthForces"=w428:T10)
        n60 = Bundle By Name(cluster=w428, "Timestamp"=w427, "XForces[12]"=w426, "YForces[100]"=w425, "ZForces[156]"=w424, "Fx"=w423, "Fy"=w422, "Fz"=w421, "Mx"=w420, "My"=w419, "Mz"=w418, "ForceMagnitude"=w417) -> (w415:T10)
        n61 = Bundle By Name(cluster=w416, "logevent_AppliedAzimuthForces"=w415) -> (w414:T1)
      }
      event User Event {
        n62 = event-data() -> ("Timestamp"=w436:dbl, "ZForces[156]"=w435:sgl[], "Fz"=w434:sgl, "Mx"=w433:sgl, "My"=w432:sgl)  [unwired: 1 in, 4 out]
        n63 = Unbundle By Name(w431) -> ("logevent_AppliedActiveOpticForces"=w437:T9)
        n64 = Bundle By Name(cluster=w437, "Timestamp"=w436, "ZForces[156]"=w435, "Fz"=w434, "Mx"=w433, "My"=w432) -> (w430:T9)
        n65 = Bundle By Name(cluster=w431, "logevent_AppliedActiveOpticForces"=w430) -> (w429:T1)
      }
      event User Event {
        n66 = event-data() -> ("Timestamp"=w451:dbl, "XForces[12]"=w450:sgl[], "YForces[100]"=w449:sgl[], "ZForces[156]"=w448:sgl[], "Fx"=w447:sgl, "Fy"=w446:sgl, "Fz"=w445:sgl, "Mx"=w444:sgl, "My"=w443:sgl, "Mz"=w442:sgl, "ForceMagnitude"=w441:sgl)  [unwired: 1 in, 4 out]
        n67 = Unbundle By Name(w440) -> ("logevent_AppliedBalanceForces"=w452:T11)
        n68 = Bundle By Name(cluster=w452, "Timestamp"=w451, "XForces[12]"=w450, "YForces[100]"=w449, "ZForces[156]"=w448, "Fx"=w447, "Fy"=w446, "Fz"=w445, "Mx"=w444, "My"=w443, "Mz"=w442, "ForceMagnitude"=w441) -> (w439:T11)
        n69 = Bundle By Name(cluster=w440, "logevent_AppliedBalanceForces"=w439) -> (w438:T1)
      }
      event User Event {
        n70 = event-data() -> ("Timestamp"=w458:dbl, "SecondaryCylinderForces[112]"=w457:i32[], "PrimaryCylinderForces[156]"=w456:i32[])  [unwired: 1 in, 4 out]
        n71 = Unbundle By Name(w455) -> ("logevent_AppliedCylinderForces"=w459:T12)
        n72 = Bundle By Name(cluster=w459, "Timestamp"=w458, "SecondaryCylinderForces[112]"=w457, "PrimaryCylinderForces[156]"=w456) -> (w454:T12)
        n73 = Bundle By Name(cluster=w455, "logevent_AppliedCylinderForces"=w454) -> (w453:T1)
      }
      event User Event {
        n74 = event-data() -> ("Timestamp"=w473:dbl, "XForces[12]"=w472:sgl[], "YForces[100]"=w471:sgl[], "ZForces[156]"=w470:sgl[], "Fx"=w469:sgl, "Fy"=w468:sgl, "Fz"=w467:sgl, "Mx"=w466:sgl, "My"=w465:sgl, "Mz"=w464:sgl, "ForceMagnitude"=w463:sgl)  [unwired: 1 in, 4 out]
        n75 = Unbundle By Name(w462) -> ("logevent_AppliedElevationForces"=w474:T13)
        n76 = Bundle By Name(cluster=w474, "Timestamp"=w473, "XForces[12]"=w472, "YForces[100]"=w471, "ZForces[156]"=w470, "Fx"=w469, "Fy"=w468, "Fz"=w467, "Mx"=w466, "My"=w465, "Mz"=w464, "ForceMagnitude"=w463) -> (w461:T13)
        n77 = Bundle By Name(cluster=w462, "logevent_AppliedElevationForces"=w461) -> (w460:T1)
      }
      event User Event {
        n78 = event-data() -> ("Timestamp"=w488:dbl, "XForces[12]"=w487:sgl[], "YForces[100]"=w486:sgl[], "ZForces[156]"=w485:sgl[], "Fx"=w484:sgl, "Fy"=w483:sgl, "Fz"=w482:sgl, "Mx"=w481:sgl, "My"=w480:sgl, "Mz"=w479:sgl, "ForceMagnitude"=w478:sgl)  [unwired: 1 in, 4 out]
        n79 = Unbundle By Name(w477) -> ("logevent_AppliedForces"=w489:T14)
        n80 = Bundle By Name(cluster=w489, "Timestamp"=w488, "XForces[12]"=w487, "YForces[100]"=w486, "ZForces[156]"=w485, "Fx"=w484, "Fy"=w483, "Fz"=w482, "Mx"=w481, "My"=w480, "Mz"=w479, "ForceMagnitude"=w478) -> (w476:T14)
        n81 = Bundle By Name(cluster=w477, "logevent_AppliedForces"=w476) -> (w475:T1)
      }
      event User Event {
        n82 = event-data() -> ("Timestamp"=w503:dbl, "XForces[12]"=w502:sgl[], "YForces[100]"=w501:sgl[], "ZForces[156]"=w500:sgl[], "Fx"=w499:sgl, "Fy"=w498:sgl, "Fz"=w497:sgl, "Mx"=w496:sgl, "My"=w495:sgl, "Mz"=w494:sgl, "ForceMagnitude"=w493:sgl)  [unwired: 1 in, 4 out]
        n83 = Unbundle By Name(w492) -> ("logevent_AppliedOffsetForces"=w504:T15)
        n84 = Bundle By Name(cluster=w504, "Timestamp"=w503, "XForces[12]"=w502, "YForces[100]"=w501, "ZForces[156]"=w500, "Fx"=w499, "Fy"=w498, "Fz"=w497, "Mx"=w496, "My"=w495, "Mz"=w494, "ForceMagnitude"=w493) -> (w491:T15)
        n85 = Bundle By Name(cluster=w492, "logevent_AppliedOffsetForces"=w491) -> (w490:T1)
      }
      event User Event {
        n86 = event-data() -> ("Timestamp"=w518:dbl, "XForces[12]"=w517:sgl[], "YForces[100]"=w516:sgl[], "ZForces[156]"=w515:sgl[], "Fx"=w514:sgl, "Fy"=w513:sgl, "Fz"=w512:sgl, "Mx"=w511:sgl, "My"=w510:sgl, "Mz"=w509:sgl, "ForceMagnitude"=w508:sgl)  [unwired: 1 in, 4 out]
        n87 = Unbundle By Name(w507) -> ("logevent_AppliedStaticForces"=w519:T16)
        n88 = Bundle By Name(cluster=w519, "Timestamp"=w518, "XForces[12]"=w517, "YForces[100]"=w516, "ZForces[156]"=w515, "Fx"=w514, "Fy"=w513, "Fz"=w512, "Mx"=w511, "My"=w510, "Mz"=w509, "ForceMagnitude"=w508) -> (w506:T16)
        n89 = Bundle By Name(cluster=w507, "logevent_AppliedStaticForces"=w506) -> (w505:T1)
      }
      event User Event {
        n90 = event-data() -> ("Timestamp"=w533:dbl, "XForces[12]"=w532:sgl[], "YForces[100]"=w531:sgl[], "ZForces[156]"=w530:sgl[], "Fx"=w529:sgl, "Fy"=w528:sgl, "Fz"=w527:sgl, "Mx"=w526:sgl, "My"=w525:sgl, "Mz"=w524:sgl, "ForceMagnitude"=w523:sgl)  [unwired: 1 in, 5 out]
        n91 = Unbundle By Name(w521) -> ("logevent_AppliedThermalForces"=w534:T17)
        n92 = Bundle By Name(cluster=w534, "Timestamp"=w533, "XForces[12]"=w532, "YForces[100]"=w531, "ZForces[156]"=w530, "Fx"=w529, "Fy"=w528, "Fz"=w527, "Mx"=w526, "My"=w525, "Mz"=w524, "ForceMagnitude"=w523) -> (w522:T17)
        n93 = Bundle By Name(cluster=w521, "logevent_AppliedThermalForces"=w522) -> (w520:T1)
      }
      event User Event {
        n94 = event-data() -> ("Timestamp"=w548:dbl, "XForces[12]"=w547:sgl[], "YForces[100]"=w546:sgl[], "ZForces[156]"=w545:sgl[], "Fx"=w544:sgl, "Fy"=w543:sgl, "Fz"=w542:sgl, "Mx"=w541:sgl, "My"=w540:sgl, "Mz"=w539:sgl, "ForceMagnitude"=w538:sgl)  [unwired: 1 in, 4 out]
        n95 = Unbundle By Name(w537) -> ("logevent_AppliedVelocityForces"=w549:T18)
        n96 = Bundle By Name(cluster=w549, "Timestamp"=w548, "XForces[12]"=w547, "YForces[100]"=w546, "ZForces[156]"=w545, "Fx"=w544, "Fy"=w543, "Fz"=w542, "Mx"=w541, "My"=w540, "Mz"=w539, "ForceMagnitude"=w538) -> (w536:T18)
        n97 = Bundle By Name(cluster=w537, "logevent_AppliedVelocityForces"=w536) -> (w535:T1)
      }
      event User Event {
        n98 = event-data() -> ("Timestamp"=w557:dbl, "ZForces[156]"=w556:sgl[], "Fz"=w555:sgl, "Mx"=w554:sgl, "My"=w553:sgl)  [unwired: 1 in, 4 out]
        n99 = Unbundle By Name(w552) -> ("logevent_RejectedAberrationForces"=w558:T19)
        n100 = Bundle By Name(cluster=w558, "Timestamp"=w557, "ZForces[156]"=w556, "Fz"=w555, "Mx"=w554, "My"=w553) -> (w551:T19)
        n101 = Bundle By Name(cluster=w552, "logevent_RejectedAberrationForces"=w551) -> (w550:T1)
      }
      event User Event {
        n102 = event-data() -> ("Timestamp"=w572:dbl, "XForces[12]"=w571:sgl[], "YForces[100]"=w570:sgl[], "ZForces[156]"=w569:sgl[], "Fx"=w568:sgl, "Fy"=w567:sgl, "Fz"=w566:sgl, "Mx"=w565:sgl, "My"=w564:sgl, "Mz"=w563:sgl, "ForceMagnitude"=w562:sgl)  [unwired: 1 in, 4 out]
        n103 = Unbundle By Name(w561) -> ("logevent_RejectedAccelerationForces"=w573:T20)
        n104 = Bundle By Name(cluster=w573, "Timestamp"=w572, "XForces[12]"=w571, "YForces[100]"=w570, "ZForces[156]"=w569, "Fx"=w568, "Fy"=w567, "Fz"=w566, "Mx"=w565, "My"=w564, "Mz"=w563, "ForceMagnitude"=w562) -> (w560:T20)
        n105 = Bundle By Name(cluster=w561, "logevent_RejectedAccelerationForces"=w560) -> (w559:T1)
      }
      event User Event {
        n106 = event-data() -> ("Timestamp"=w581:dbl, "ZForces[156]"=w580:sgl[], "Fz"=w579:sgl, "Mx"=w578:sgl, "My"=w577:sgl)  [unwired: 1 in, 4 out]
        n107 = Unbundle By Name(w576) -> ("logevent_RejectedActiveOpticForces"=w582:T21)
        n108 = Bundle By Name(cluster=w582, "Timestamp"=w581, "ZForces[156]"=w580, "Fz"=w579, "Mx"=w578, "My"=w577) -> (w575:T21)
        n109 = Bundle By Name(cluster=w576, "logevent_RejectedActiveOpticForces"=w575) -> (w574:T1)
      }
      event User Event {
        n110 = event-data() -> ("Timestamp"=w596:dbl, "XForces[12]"=w595:sgl[], "YForces[100]"=w594:sgl[], "ZForces[156]"=w593:sgl[], "Fx"=w592:sgl, "Fy"=w591:sgl, "Fz"=w590:sgl, "Mx"=w589:sgl, "My"=w588:sgl, "Mz"=w587:sgl, "ForceMagnitude"=w586:sgl)  [unwired: 1 in, 4 out]
        n111 = Unbundle By Name(w585) -> ("logevent_RejectedAzimuthForces"=w597:T22)
        n112 = Bundle By Name(cluster=w597, "Timestamp"=w596, "XForces[12]"=w595, "YForces[100]"=w594, "ZForces[156]"=w593, "Fx"=w592, "Fy"=w591, "Fz"=w590, "Mx"=w589, "My"=w588, "Mz"=w587, "ForceMagnitude"=w586) -> (w584:T22)
        n113 = Bundle By Name(cluster=w585, "logevent_RejectedAzimuthForces"=w584) -> (w583:T1)
      }
      event User Event {
        n114 = event-data() -> ("Timestamp"=w611:dbl, "XForces[12]"=w610:sgl[], "YForces[100]"=w609:sgl[], "ZForces[156]"=w608:sgl[], "Fx"=w607:sgl, "Fy"=w606:sgl, "Fz"=w605:sgl, "Mx"=w604:sgl, "My"=w603:sgl, "Mz"=w602:sgl, "ForceMagnitude"=w601:sgl)  [unwired: 1 in, 4 out]
        n115 = Unbundle By Name(w600) -> ("logevent_RejectedBalanceForces"=w612:T23)
        n116 = Bundle By Name(cluster=w612, "Timestamp"=w611, "XForces[12]"=w610, "YForces[100]"=w609, "ZForces[156]"=w608, "Fx"=w607, "Fy"=w606, "Fz"=w605, "Mx"=w604, "My"=w603, "Mz"=w602, "ForceMagnitude"=w601) -> (w599:T23)
        n117 = Bundle By Name(cluster=w600, "logevent_RejectedBalanceForces"=w599) -> (w598:T1)
      }
      event User Event {
        n118 = event-data() -> ("Timestamp"=w618:dbl, "SecondaryCylinderForces[112]"=w617:i32[], "PrimaryCylinderForces[156]"=w616:i32[])  [unwired: 1 in, 4 out]
        n119 = Unbundle By Name(w615) -> ("logevent_RejectedCylinderForces"=w619:T24)
        n120 = Bundle By Name(cluster=w619, "Timestamp"=w618, "SecondaryCylinderForces[112]"=w617, "PrimaryCylinderForces[156]"=w616) -> (w614:T24)
        n121 = Bundle By Name(cluster=w615, "logevent_RejectedCylinderForces"=w614) -> (w613:T1)
      }
      event User Event {
        n122 = event-data() -> ("Timestamp"=w633:dbl, "XForces[12]"=w632:sgl[], "YForces[100]"=w631:sgl[], "ZForces[156]"=w630:sgl[], "Fx"=w629:sgl, "Fy"=w628:sgl, "Fz"=w627:sgl, "Mx"=w626:sgl, "My"=w625:sgl, "Mz"=w624:sgl, "ForceMagnitude"=w623:sgl)  [unwired: 1 in, 4 out]
        n123 = Unbundle By Name(w622) -> ("logevent_RejectedElevationForces"=w634:T25)
        n124 = Bundle By Name(cluster=w634, "Timestamp"=w633, "XForces[12]"=w632, "YForces[100]"=w631, "ZForces[156]"=w630, "Fx"=w629, "Fy"=w628, "Fz"=w627, "Mx"=w626, "My"=w625, "Mz"=w624, "ForceMagnitude"=w623) -> (w621:T25)
        n125 = Bundle By Name(cluster=w622, "logevent_RejectedElevationForces"=w621) -> (w620:T1)
      }
      event User Event {
        n126 = event-data() -> ("Timestamp"=w648:dbl, "XForces[12]"=w647:sgl[], "YForces[100]"=w646:sgl[], "ZForces[156]"=w645:sgl[], "Fx"=w644:sgl, "Fy"=w643:sgl, "Fz"=w642:sgl, "Mx"=w641:sgl, "My"=w640:sgl, "Mz"=w639:sgl, "ForceMagnitude"=w638:sgl)  [unwired: 1 in, 4 out]
        n127 = Unbundle By Name(w637) -> ("logevent_RejectedForces"=w649:T26)
        n128 = Bundle By Name(cluster=w649, "Timestamp"=w648, "XForces[12]"=w647, "YForces[100]"=w646, "ZForces[156]"=w645, "Fx"=w644, "Fy"=w643, "Fz"=w642, "Mx"=w641, "My"=w640, "Mz"=w639, "ForceMagnitude"=w638) -> (w636:T26)
        n129 = Bundle By Name(cluster=w637, "logevent_RejectedForces"=w636) -> (w635:T1)
      }
      event User Event {
        n130 = event-data() -> ("Timestamp"=w653:dbl, "XForces[12]"=w654:sgl[], "YForces[100]"=w655:sgl[], "ZForces[156]"=w656:sgl[], "Fx"=w657:sgl, "Fy"=w658:sgl, "Fz"=w659:sgl, "Mx"=w660:sgl, "My"=w661:sgl, "Mz"=w662:sgl, "ForceMagnitude"=w663:sgl)  [unwired: 1 in, 4 out]
        n131 = Unbundle By Name(w652) -> ("logevent_RejectedOffsetForces"=w664:T27)
        n132 = Bundle By Name(cluster=w664, "Timestamp"=w653, "XForces[12]"=w654, "YForces[100]"=w655, "ZForces[156]"=w656, "Fx"=w657, "Fy"=w658, "Fz"=w659, "Mx"=w660, "My"=w661, "Mz"=w662, "ForceMagnitude"=w663) -> (w651:T27)
        n133 = Bundle By Name(cluster=w652, "logevent_RejectedOffsetForces"=w651) -> (w650:T1)
      }
      event User Event {
        n134 = event-data() -> ("Timestamp"=w678:dbl, "XForces[12]"=w677:sgl[], "YForces[100]"=w676:sgl[], "ZForces[156]"=w675:sgl[], "Fx"=w674:sgl, "Fy"=w673:sgl, "Fz"=w672:sgl, "Mx"=w671:sgl, "My"=w670:sgl, "Mz"=w669:sgl, "ForceMagnitude"=w668:sgl)  [unwired: 1 in, 4 out]
        n135 = Unbundle By Name(w667) -> ("logevent_RejectedThermalForces"=w679:T29)
        n136 = Bundle By Name(cluster=w679, "Timestamp"=w678, "XForces[12]"=w677, "YForces[100]"=w676, "ZForces[156]"=w675, "Fx"=w674, "Fy"=w673, "Fz"=w672, "Mx"=w671, "My"=w670, "Mz"=w669, "ForceMagnitude"=w668) -> (w666:T29)
        n137 = Bundle By Name(cluster=w667, "logevent_RejectedThermalForces"=w666) -> (w665:T1)
      }
      event User Event {
        n138 = event-data() -> ("Timestamp"=w693:dbl, "XForces[12]"=w692:sgl[], "YForces[100]"=w691:sgl[], "ZForces[156]"=w690:sgl[], "Fx"=w689:sgl, "Fy"=w688:sgl, "Fz"=w687:sgl, "Mx"=w686:sgl, "My"=w685:sgl, "Mz"=w684:sgl, "ForceMagnitude"=w683:sgl)  [unwired: 1 in, 4 out]
        n139 = Unbundle By Name(w682) -> ("logevent_RejectedVelocityForces"=w694:T30)
        n140 = Bundle By Name(cluster=w694, "Timestamp"=w693, "XForces[12]"=w692, "YForces[100]"=w691, "ZForces[156]"=w690, "Fx"=w689, "Fy"=w688, "Fz"=w687, "Mx"=w686, "My"=w685, "Mz"=w684, "ForceMagnitude"=w683) -> (w681:T30)
        n141 = Bundle By Name(cluster=w682, "logevent_RejectedVelocityForces"=w681) -> (w680:T1)
      }
    }
    n142 = flat-sequence {
      tunnel: w154 -> [w223]
      tunnel: [w223] -> w97
      frame #0 {
        n143 = local write "FA Data And Events"(w223) -> ()
      }
    }
    n144 = Unbundle By Name(w97) -> ("logevent_ForceActuatorWarning"=w153:T6)
    n145 = Unbundle By Name(w153) -> ("AnyWarning"=→"Any Warning":bool, "AnyMajorFault"=→"Any Major Fault":bool, "AnyMinorFault"=→"Any Minor Fault":bool, "AnyFaultOverride"=→"Any Fault Override":bool, "AnyMainCalibrationError"=→"Any Main Calibration Error":bool, "AnyBackupCalibrationError"=→"Any Backup Calibration Error":bool, "AnyMezzanineError"=→"Any Mezzanine Error":bool, "AnyMezzanineBootloaderActive"=→"Any Mezzanine Bootloader Active":bool, "AnyUniqueIdCRCError"=→"Any Unique Id CRC Error":bool, "AnyApplicationTypeMismatch"=→"Any Application Type Mismatch":bool, "AnyApplicationMissing"=→"Any Application Missing":bool, "AnyApplicationCRCMismatch"=→"Any Application CRC Missing":bool, "AnyOneWireMissing"=→"Any One Wire Missing":bool, "AnyOneWire1Mismatch"=→"Any One Wire 1 Mismatch":bool, "AnyOneWire2Mismatch"=→"Any One Wire 2 Mismatch":bool, "AnyWatchdogReset"=→"Any Watchdog Reset":bool, "AnyBrownOut"=→"Any Brown Out":bool, "AnyEventTrapReset"=→"Any Event Trap Reset":bool, "AnySSRPowerFault"=→"Any SSR Power Fault":bool, "AnyAuxPowerFault"=→"Any Aux Power Fault":bool, "AnyMezzaninePowerFault"=→"Any Mezzanine Power Fault":bool, "AnyMezzanineCurrentAmp1Fault"=→"Any Mezzanine Current Amp 1 Fault":bool, "AnyMezzanineCurrentAmp2Fault"=→"Any Mezzanine Current Amp 2 Fault":bool, "AnyMezzanineUniqueIdCRCError"=→"Any Mezzanine Unique Id CRC Error":bool, "AnyMezzanineMainCalibrationError"=→"Any Mezzanine Main Calibration Error":bool, "AnyMezzanineBackupCalibrationError"=→"Any Mezzanine Backup Calibration Error":bool, "AnyMezzanineEventTrapReset"=→"Any Mezzanine Event Trap Reset":bool, "AnyMezzanineApplicationMissing"=→"Any Mezzanine Application Missing":bool, "AnyMezzanineApplicationCRCMismatch"=→"Any Mezzanine Application CRC Missing":bool, "AnyILCFault"=→"Any ILC Fault":bool, "AnyBroadcastCounterWarning"=→"Any Broadcast Counter Warning":bool)  [unwired: 32 out]
    n146 = Unbundle By Name(w97) -> ("logevent_ForceActuatorState"=w121:T5)
    n147 = Unbundle By Name(w97) -> ("logevent_ForceActuatorForceWarning"=w108:T3)
    n148 = Unbundle By Name(w121) -> ("SlewFlag"=→"Slew Flag":bool, "StaticForcesApplied"=→"Static Forces Applied":bool, "ElevationForcesApplied"=→"Elevation Forces Applied":bool, "AzimuthForcesApplied"=→"Azimuth Forces Applied":bool, "ThermalForcesApplied"=→"Thermal Forces Applied":bool, "OffsetForcesApplied"=→"Offset Forces Applied":bool, "AccelerationForcesApplied"=→"Acceleration Forces Applied":bool, "VelocityForcesApplied"=→"Velocity Forces Applied":bool, "ActiveOpticForcesApplied"=→"Active Optic Forces Applied":bool, "AberrationForcesApplied"=→"Aberration Forces Applied":bool, "BalanceForcesApplied"=→"Balance Forces Applied":bool, "SupportPercentage"=→"Support %":sgl)  [unwired: 3 out]
    n149 = control-ref of="FA Data And Events"() -> (w94:refnum<vi>)
    n150 = Unbundle By Name(w108) -> ("AnyWarning"=→"Any Force Warning":bool, "AnyPrimaryAxisMeasuredForceWarning"=→"Any Primary Axis Measured Force Warning":bool, "AnySecondaryAxisMeasuredForceWarning"=→"Any Secondary Axis Measured Force Warning":bool, "AnyPrimaryAxisFollowingErrorWarning"=→"Any Primary Axis Following Error Warning":bool, "AnySecondaryAxisFollowingErrorWarning"=→"Any Secondary Axis Following Error Warning":bool)  [unwired: 6 out]
    n151 = call "Get FA Data.vi"("Clust Refnum"=w94, "FA Chosen Data Type"="Data Type") -> ("error out"=w100:errorcluster, "ControlRefNums"=w99:refnum<vi>[])  [unwired: 8 in]
    n152 = Merge Errors(w100, w96) -> (w98:errorcluster)
    n153 = for {
      tunnel: w99 -> [w167] mode=indexing
      shift-right: [w160] -> w95
      shift-left: w98 -> [w166]
      shift-right: [w162] -> _
      shift-left: FALSE -> [w163]
      n154 = property class="Ctl"(reference=w167, error in=w166) -> (reference out=w169:refnum<vi>, error out=w170:errorcluster, "Label.Text"=w164:string)
      n155 = property class="Ctl"(reference=w169, error in=w170) -> (reference out=w159:refnum<vi>, error out=w168:errorcluster, "Value"=w165:variant)
      n156 = case shown="\"Mx\"" w164 {
        tunnel: w165 -> [_ w176 w184 w192 w197 w203 w209 w215 w221]
        tunnel: w168 -> [w172 w175 w185 w190 w196 w202 w208 w214 w220]
        tunnel: [w172 w174 w186 w189 w194 w200 w207 w213 w219] -> w161
        tunnel: w163 -> [w171 _ _ _ _ _ _ _ _]
        tunnel: [w171 TRUE TRUE TRUE TRUE TRUE TRUE TRUE TRUE] -> w162
        frame "", Default {
        }
        frame "Timestamp" {
          n157 = Variant To Data(error in=w175, type=0.0, Variant=w176) -> (data=w179:dbl, error out=w174:errorcluster)
          n158 = call "Get Timestamp Cushion.vi"("DoubleTimestampRepresentation"=w179) -> ("TimestampCushion"=w177:dbl)  [unwired: 10 in]
          n159 = To Time Stamp(1:w177) -> (0:→"Timestamp":timestamp)
        }
        frame "Fx" {
          n160 = Variant To Data(error in=w185, type=sgl 0.0, Variant=w184) -> (data=→"Fx":sgl, error out=w186:errorcluster)
        }
        frame "Fy" {
          n161 = Variant To Data(error in=w190, type=sgl 0.0, Variant=w192) -> (data=→"Fy":sgl, error out=w189:errorcluster)
        }
        frame "Fz" {
          n162 = Variant To Data(error in=w196, type=sgl 0.0, Variant=w197) -> (data=→"Fz":sgl, error out=w194:errorcluster)
        }
        frame "Mx" {
          n163 = Variant To Data(error in=w202, type=sgl 0.0, Variant=w203) -> (data=→"Mx":sgl, error out=w200:errorcluster)
        }
        frame "My" {
          n164 = Variant To Data(error in=w208, type=sgl 0.0, Variant=w209) -> (data=→"My":sgl, error out=w207:errorcluster)
        }
        frame "Mz" {
          n165 = Variant To Data(error in=w214, type=sgl 0.0, Variant=w215) -> (data=→"Mz":sgl, error out=w213:errorcluster)
        }
        frame "ForceMagnitude" {
          n166 = Variant To Data(error in=w220, type=sgl 0.0, Variant=w221) -> (data=→"Force Magnitude":sgl, error out=w219:errorcluster)
        }
      }
      n167 = Close Reference(reference=w159, error in (no error)=w161) -> (error out=w160:errorcluster)
    }
  }
  n168 = Unregister For Events(event registration refnum=w15, error in=w14) -> (error out=w13:errorcluster)
  n169 = call <vilib>:"Simple Error Handler.vi"("error in (no error)"=w13) -> ()  [unwired: 4 in, 5 out]
